vi "create_pb_arrayofarrays_synth_v2012.vi"(0 "PulseBlaster Array of Arrays":T12(array[cluster])=[{"Data Field"=0, "Delay"=0.005, "OP code"=8, "Output Bits"=[FALSE, TRUE, FALSE, FALSE, FALSE, FALSE, FALSE, FALSE, FALSE, FALSE, FALSE, FALSE, TRUE, FALSE, FALSE, FALSE, FALSE, FALSE, FALSE, FALSE, FALSE, FALSE, FALSE, FALSE], "String"="cool mot coils"}, {"Data Field"=300, "Delay"=0.000999, "OP code"=2, "Output Bits"=[TRUE, TRUE, TRUE, TRUE, FALSE, FALSE, TRUE, FALSE, FALSE, TRUE, FALSE, FALSE, TRUE, TRUE, FALSE, TRUE, TRUE, FALSE, FALSE, FALSE, FALSE, FALSE, FALSE, FALSE], "String"="mot load loop"}, {"Data Field"=1, "Delay"=1e-06, "OP code"=3, "Output Bits"=[TRUE, TRUE, TRUE, TRUE, FALSE, FALSE, TRUE, FALSE, FALSE, TRUE, FALSE, FALSE, TRUE, TRUE, FALSE, TRUE, TRUE, FALSE, FALSE, FALSE, FALSE, FALSE, FALSE, FALSE, FALSE], "String"=""}, {"Data Field"=0, "Delay"=0.001, "OP code"=0, "Output Bits"=[TRUE, TRUE, TRUE, TRUE, FALSE, FALSE, TRUE, FALSE, FALSE, TRUE, FALSE, FALSE, TRUE, TRUE, FALSE, TRUE, TRUE, FALSE, FALSE, FALSE, FALSE, FALSE, FALSE, FALSE], "String"=""}, {"Data Field"=2, "Delay"=0.000999, "OP code"=2, "Output Bits"=[TRUE, TRUE, TRUE, TRUE, FALSE, FALSE, TRUE, FALSE, FALSE, TRUE, FALSE, FALSE, TRUE, TRUE, FALSE, TRUE, TRUE, FALSE, FALSE, FALSE, FALSE, FALSE, FALSE, FALSE], "String"="mot decay loop"}, {"Data Field"=4, "Delay"=1e-06, "OP code"=3, "Output Bits"=[TRUE, TRUE, TRUE, TRUE, FALSE, FALSE, TRUE, FALSE, FALSE, TRUE, FALSE, FALSE, TRUE, TRUE, FALSE, TRUE, TRUE, FALSE, FALSE, FALSE, FALSE, FALSE, FALSE, FALSE], "String"=""}, {"Data Field"=0, "Delay"=0.000908, "OP code"=0, "Output Bits"=[TRUE, TRUE, TRUE, TRUE, FALSE, FALSE, TRUE, FALSE, FALSE, TRUE, FALSE, FALSE, TRUE, TRUE, FALSE, TRUE, TRUE, FALSE, FALSE, FALSE, FALSE, FALSE, FALSE, FALSE], "String"=""}, {"Data Field"=0, "Delay"=0.00865, "OP code"=0, "Output Bits"=[TRUE, TRUE, TRUE, TRUE, FALSE, FALSE, TRUE, FALSE, FALSE, TRUE, FALSE, FALSE, TRUE, TRUE, FALSE, TRUE, TRUE, FALSE, FALSE, FALSE, FALSE, FALSE, FALSE, FALSE], "String"=""}, {"Data Field"=0, "Delay"=0.004, "OP code"=0, "Output Bits"=[TRUE, TRUE, FALSE, TRUE, FALSE, FALSE, TRUE, FALSE, FALSE, TRUE, FALSE, FALSE, TRUE, TRUE, FALSE, TRUE, TRUE, FALSE, FALSE, FALSE, FALSE, FALSE, FALSE, FALSE], "String"=""}, {"Data Field"=0, "Delay"=0.0045, "OP code"=0, "Output Bits"=[TRUE, TRUE, FALSE, TRUE, FALSE, FALSE, TRUE, FALSE, FALSE, TRUE, FALSE, FALSE, TRUE, FALSE, FALSE, FALSE, TRUE, FALSE, FALSE, FALSE, FALSE, FALSE, FALSE, FALSE], "String"="Blue MOT Cooling Time"}, {"Data Field"=0, "Delay"=0.05, "OP code"=0, "Output Bits"=[FALSE, TRUE, FALSE, FALSE, FALSE, FALSE, FALSE, FALSE, FALSE, TRUE, TRUE, FALSE, TRUE, FALSE, FALSE, FALSE, FALSE, FALSE, FALSE, FALSE, FALSE, FALSE, FALSE, FALSE], "String"="Red MOT Cooling Time =="}, {"Data Field"=0, "Delay"=0.01, "OP code"=0, "Output Bits"=[FALSE, TRUE, FALSE, FALSE, FALSE, FALSE, FALSE, FALSE, FALSE, FALSE, FALSE, FALSE, FALSE, FALSE, FALSE, FALSE, FALSE, FALSE, FALSE, FALSE, FALSE, FALSE, FALSE, FALSE], "String"="PAS Beam with RED MOT            DELAY TIME BEFORE INTERAC"}, {"Data Field"=0, "Delay"=0.005, "OP code"=0, "Output Bits"=[FALSE, TRUE, FALSE, FALSE, FALSE, FALSE, FALSE, FALSE, FALSE, FALSE, FALSE, FALSE, FALSE, FALSE, FALSE, FALSE, TRUE, FALSE, FALSE, FALSE, FALSE, FALSE, FALSE, FALSE], "String"="image 12 delay (150n=90ndelay) INTERAC TIME"}, {"Data Field"=0, "Delay"=5e-05, "OP code"=0, "Output Bits"=[FALSE, TRUE, FALSE, FALSE, FALSE, FALSE, FALSE, FALSE, FALSE, FALSE, FALSE, FALSE, FALSE, FALSE, FALSE, FALSE, TRUE, TRUE, FALSE, FALSE, FALSE, FALSE, FALSE, FALSE], "String"="image beam on"}, {"Data Field"=0, "Delay"=0.0002, "OP code"=0, "Output Bits"=[FALSE, FALSE, FALSE, FALSE, FALSE, TRUE, FALSE, FALSE, FALSE, FALSE, FALSE, FALSE, FALSE, FALSE, FALSE, FALSE, TRUE, TRUE, FALSE, FALSE, FALSE, FALSE, FALSE, FALSE], "String"="camera minimum exposure time"}, {"Data Field"=0, "Delay"=0.07, "OP code"=0, "Output Bits"=[FALSE, FALSE, FALSE, FALSE, FALSE, FALSE, FALSE, FALSE, FALSE, FALSE, FALSE, FALSE, FALSE, FALSE, FALSE, FALSE, FALSE, TRUE, FALSE, FALSE, FALSE, FALSE, FALSE, FALSE], "String"="PixelFly Readout 1"}, {"Data Field"=0, "Delay"=0.005, "OP code"=0, "Output Bits"=[FALSE, FALSE, FALSE, FALSE, FALSE, FALSE, FALSE, FALSE, FALSE, FALSE, FALSE, FALSE, FALSE, FALSE, FALSE, FALSE, TRUE, TRUE, FALSE, FALSE, FALSE, FALSE, FALSE, FALSE], "String"="shutter opening time"}, {"Data Field"=0, "Delay"=0.0002, "OP code"=0, "Output Bits"=[FALSE, FALSE, FALSE, FALSE, FALSE, TRUE, FALSE, FALSE, FALSE, FALSE, FALSE, FALSE, FALSE, FALSE, FALSE, FALSE, TRUE, TRUE, FALSE, FALSE, FALSE, FALSE, FALSE, FALSE], "String"="Pixelfly exposure 2"}, {"Data Field"=0, "Delay"=0.07, "OP code"=0, "Output Bits"=[FALSE, FALSE, FALSE, FALSE, FALSE, FALSE, FALSE, FALSE, FALSE, FALSE, FALSE, FALSE, FALSE, FALSE, FALSE, FALSE, FALSE, FALSE, FALSE, FALSE, FALSE, FALSE, FALSE, FALSE], "String"="PixelFly readout 2"}, {"Data Field"=0, "Delay"=0.001, "OP code"=6, "Output Bits"=[FALSE, TRUE, TRUE, TRUE, FALSE, FALSE, FALSE, FALSE, FALSE, FALSE, FALSE, FALSE, TRUE, TRUE, FALSE, TRUE, FALSE, FALSE, FALSE, FALSE, FALSE, FALSE, FALSE, FALSE], "String"=""}] {"OP code" items=["Continue", "Stop", "Loop", "End Loop", "Jump", "Return", "Go To", "Long Delay", "Wait"]; "Delay" format="%.3p"}, 1 "6713 Write":dbl[](array[numeric])=[1.0, 4.0, 0.5, 6.5, 0.0, 9.58, 3.5, 0.5] format="%.3f", 2 "Arbitrary Waveform Array of Channels":T7(array[cluster])=[[{"AC Frequency (kHz)"=40.0, " Initial AC Ampl. (p-p/2)"=0.0, "Final AC Ampl."=0.0, "Initial DC Value"=-0.25, "Final DC Value"=0.05, "Constant"=165.3, "Gamma AC"=1.0, "String"="Channel 0 A", "Gamma DC"=1.0}, {"AC Frequency (kHz)"=40.0, " Initial AC Ampl. (p-p/2)"=0.0, "Final AC Ampl."=0.0, "Initial DC Value"=0.0, "Final DC Value"=0.0, "Constant"=165.2, "Gamma AC"=1.0, "String"="Channel 0 B", "Gamma DC"=1.0}, {"AC Frequency (kHz)"=40.0, " Initial AC Ampl. (p-p/2)"=0.0, "Final AC Ampl."=0.0, "Initial DC Value"=0.0, "Final DC Value"=0.0, "Constant"=163.20000000000002, "Gamma AC"=1.0, "String"="Channel 0 C", "Gamma DC"=1.0}], [{"AC Frequency (kHz)"=10.0, " Initial AC Ampl. (p-p/2)"=5.0, "Final AC Ampl."=0.0, "Initial DC Value"=0.2, "Final DC Value"=0.14, "Constant"=0.25, "Gamma AC"=1.0, "String"="Channel 1 A", "Gamma DC"=1.0}, {"AC Frequency (kHz)"=10.0, " Initial AC Ampl. (p-p/2)"=5.0, "Final AC Ampl."=0.0, "Initial DC Value"=0.1, "Final DC Value"=0.1, "Constant"=0.25, "Gamma AC"=1.0, "String"="Channel 1 B", "Gamma DC"=1.0}, {"AC Frequency (kHz)"=10.0, " Initial AC Ampl. (p-p/2)"=0.0, "Final AC Ampl."=0.0, "Initial DC Value"=0.0, "Final DC Value"=0.0, "Constant"=0.25, "Gamma AC"=1.0, "String"="Channel 1 C", "Gamma DC"=1.0}], [{"AC Frequency (kHz)"=10.0, " Initial AC Ampl. (p-p/2)"=0.0, "Final AC Ampl."=0.0, "Initial DC Value"=0.007, "Final DC Value"=0.04, "Constant"=0.0, "Gamma AC"=1.0, "String"="Channel 2 A", "Gamma DC"=1.0}, {"AC Frequency (kHz)"=10.0, " Initial AC Ampl. (p-p/2)"=0.0, "Final AC Ampl."=0.0, "Initial DC Value"=0.5, "Final DC Value"=0.5, "Constant"=0.0, "Gamma AC"=1.0, "String"="Channel 2 B", "Gamma DC"=1.0}, {"AC Frequency (kHz)"=10.0, " Initial AC Ampl. (p-p/2)"=0.0, "Final AC Ampl."=0.0, "Initial DC Value"=0.0, "Final DC Value"=0.0, "Constant"=0.0, "Gamma AC"=1.0, "String"="Channel 2 C", "Gamma DC"=1.0}], [{"AC Frequency (kHz)"=10.0, " Initial AC Ampl. (p-p/2)"=0.0, "Final AC Ampl."=0.0, "Initial DC Value"=1.0, "Final DC Value"=1.0, "Constant"=199.2, "Gamma AC"=1.0, "String"="Channel 3 A", "Gamma DC"=1.0}, {"AC Frequency (kHz)"=10.0, " Initial AC Ampl. (p-p/2)"=0.0, "Final AC Ampl."=0.0, "Initial DC Value"=1.0, "Final DC Value"=1.0, "Constant"=199.2, "Gamma AC"=1.0, "String"="Channel 3 B", "Gamma DC"=1.0}, {"AC Frequency (kHz)"=10.0, " Initial AC Ampl. (p-p/2)"=0.0, "Final AC Ampl."=0.0, "Initial DC Value"=1.0, "Final DC Value"=1.0, "Constant"=199.2, "Gamma AC"=1.0, "String"="Channel 3 C", "Gamma DC"=1.0}], [{"AC Frequency (kHz)"=10.0, " Initial AC Ampl. (p-p/2)"=0.0, "Final AC Ampl."=0.0, "Initial DC Value"=-0.1, "Final DC Value"=-0.04, "Constant"=199.2, "Gamma AC"=1.0, "String"="Channel 4 A", "Gamma DC"=1.0}, {"AC Frequency (kHz)"=10.0, " Initial AC Ampl. (p-p/2)"=0.0, "Final AC Ampl."=0.0, "Initial DC Value"=-0.1, "Final DC Value"=-0.04, "Constant"=199.2, "Gamma AC"=1.0, "String"="Channel 4 B", "Gamma DC"=1.0}, {"AC Frequency (kHz)"=10.0, " Initial AC Ampl. (p-p/2)"=0.0, "Final AC Ampl."=0.0, "Initial DC Value"=-0.1, "Final DC Value"=-0.04, "Constant"=199.2, "Gamma AC"=1.0, "String"="Channel 4 C", "Gamma DC"=1.0}], [{"AC Frequency (kHz)"=10.0, " Initial AC Ampl. (p-p/2)"=0.0, "Final AC Ampl."=0.0, "Initial DC Value"=-0.1, "Final DC Value"=-0.04, "Constant"=199.2, "Gamma AC"=1.0, "String"="Channel 5 A", "Gamma DC"=1.0}, {"AC Frequency (kHz)"=10.0, " Initial AC Ampl. (p-p/2)"=0.0, "Final AC Ampl."=0.0, "Initial DC Value"=-0.1, "Final DC Value"=-0.04, "Constant"=199.2, "Gamma AC"=1.0, "String"="Channel 5 B", "Gamma DC"=1.0}, {"AC Frequency (kHz)"=10.0, " Initial AC Ampl. (p-p/2)"=0.0, "Final AC Ampl."=0.0, "Initial DC Value"=-0.1, "Final DC Value"=-0.04, "Constant"=199.2, "Gamma AC"=1.0, "String"="Channel 5 C", "Gamma DC"=1.0}], [{"AC Frequency (kHz)"=10.0, " Initial AC Ampl. (p-p/2)"=0.0, "Final AC Ampl."=0.0, "Initial DC Value"=-0.1, "Final DC Value"=-0.04, "Constant"=199.2, "Gamma AC"=1.0, "String"="Channel 6 A", "Gamma DC"=1.0}, {"AC Frequency (kHz)"=10.0, " Initial AC Ampl. (p-p/2)"=0.0, "Final AC Ampl."=0.0, "Initial DC Value"=-0.1, "Final DC Value"=-0.04, "Constant"=199.2, "Gamma AC"=1.0, "String"="Channel 6 B", "Gamma DC"=1.0}, {"AC Frequency (kHz)"=10.0, " Initial AC Ampl. (p-p/2)"=0.0, "Final AC Ampl."=0.0, "Initial DC Value"=-0.1, "Final DC Value"=-0.04, "Constant"=199.2, "Gamma AC"=1.0, "String"="Channel 6 C", "Gamma DC"=1.0}], [{"AC Frequency (kHz)"=10.0, " Initial AC Ampl. (p-p/2)"=0.0, "Final AC Ampl."=0.0, "Initial DC Value"=-0.1, "Final DC Value"=-0.04, "Constant"=199.2, "Gamma AC"=1.0, "String"="Channel 7 A", "Gamma DC"=1.0}, {"AC Frequency (kHz)"=10.0, " Initial AC Ampl. (p-p/2)"=0.0, "Final AC Ampl."=0.0, "Initial DC Value"=-0.1, "Final DC Value"=-0.04, "Constant"=199.2, "Gamma AC"=1.0, "String"="Channel 7 B", "Gamma DC"=1.0}, {"AC Frequency (kHz)"=10.0, " Initial AC Ampl. (p-p/2)"=0.0, "Final AC Ampl."=0.0, "Initial DC Value"=-0.1, "Final DC Value"=-0.04, "Constant"=199.2, "Gamma AC"=1.0, "String"="Channel 7 C", "Gamma DC"=1.0}]] {"Gamma DC" format="%.2f"; "Gamma AC" format="%.2f"; "Constant" min=0.0 max=240.0 format="%.3f"; "Final DC Value" format="%.3f"; "Initial DC Value" format="%.3f"; "Final AC Ampl." format="%.3f"; "Initial AC Ampl. (p-p/2)" format="%.3f"; "AC Frequency (kHz)" format="%.2f"}, 3 "Interval Lengths (ms)":dbl[](array[numeric])=[55.0, 45.0, 1.0] format="%.3f", 4 "Intervals: ON or OFF?":bool[](array[boolean])=[TRUE, FALSE, FALSE], 5 "Waveform Change Parameters":T8={"Channel to Change"=0, "Interval to Change"=1, "Waveform Parameter\nto Change"=8} {"Waveform Parameter\nto Change" items=["Constant", "Initial DC", "Final DC", "Gamma DC", "AC Frequency", "Initial AC", "Gamma AC", "Final AC", "Interval Length"]; "Interval to Change" items=["A", "B", "C", "D", "E"]}, 6 "Arrays":T2={"Logarithmic Array"={"Initial Value"=1, "Fineness Factor"=1, "Number of Values"=10, "Generate Logarithmic\nArray?"=FALSE}, "Generated Array"={"Step Size"=-0.03, "Use generated\nDAC array values?"=FALSE, "Number of DAC Array\nValues to Generate"=67, "Initial Value for DAC"=[1.0]}} {"Generated Array"."Initial Value for DAC" format="%.2f"; "Generated Array"."Step Size" format="%.4f"}, 7 "Parameters to Change":T10={"PB parameter to change"=0, "Column of\nData to Change\n(0, 1, 2, ....)"=0, "Column of\nDelay to Change\n(0, 1, 2, ....)"=11, "6713 DAC Ch\nto Change"=7, "column for waveform\n(red mot cooling)"=10, "# of PB arrays"=1, "column for waveform\n(dipole trap loading)"=10, "Power\nSupply\nChannel"=1} {"Power\nSupply\nChannel" min=1 max=2; "PB parameter to change" min=0 max=8}, 8 "Synth":T3={"Table Mode On?"=FALSE, "Synth"=[{"AC Frequency (kHz)"=0.0, " Initial AC Ampl. (p-p/2)"=0.4, "Final AC Ampl."=0.4, "Frequency"=4.0, "Phase (rad)"=0.0, "Voltage (%)"=0.0, "Gamma AC"=1.0, "String"="Channel 0 A", "Blanck"=0.0}, {"AC Frequency (kHz)"=0.0, " Initial AC Ampl. (p-p/2)"=0.4, "Final AC Ampl."=0.4, "Frequency"=4.0, "Phase (rad)"=0.0, "Voltage (%)"=0.0, "Gamma AC"=1.0, "String"="Channel 0 B", "Blanck"=-0.3}, {"AC Frequency (kHz)"=0.0, " Initial AC Ampl. (p-p/2)"=0.4, "Final AC Ampl."=0.4, "Frequency"=1.0, "Phase (rad)"=0.0, "Voltage (%)"=2.0, "Gamma AC"=1.0, "String"="Channel 0 C", "Blanck"=0.0}, {"AC Frequency (kHz)"=0.0, " Initial AC Ampl. (p-p/2)"=0.4, "Final AC Ampl."=0.4, "Frequency"=7.0, "Phase (rad)"=1.0, "Voltage (%)"=2.0, "Gamma AC"=1.0, "String"="Channel 0 D", "Blanck"=1.4}, {"AC Frequency (kHz)"=0.0, " Initial AC Ampl. (p-p/2)"=0.0, "Final AC Ampl."=0.0, "Frequency"=0.6, "Phase (rad)"=1.0, "Voltage (%)"=1.0, "Gamma AC"=0.0, "String"="Channel 0 E", "Blanck"=0.2}]} {"Synth"."Blanck" format="%.2f"; "Synth"."Gamma AC" format="%.2f"; "Synth"."Voltage (%)" min=0.0 max=100.0 step=1.0; "Synth"."Phase (rad)" min=0.0 max=6.383118 format="%#_4f"; "Synth"."Frequency" min=0.0 max=10.0 format="%.7f"; "Synth"."Final AC Ampl." format="%.3f"; "Synth"."Initial AC Ampl. (p-p/2)" format="%.3f"; "Synth"."AC Frequency (kHz)" format="%.2f"}, 9 "dac offset":dbl format="%.2f", 11 "DAC Array":dbl[](array[numeric])=[0.05, 0.1, 0.15, 0.2, 0.25, 0.3, 0.35, 0.4, 0.45, 0.5, 9.6, 0.24, 0.26, 5.28, 0.3, 0.32, 0.34, 0.36, 0.38, 0.4, 5.0, 5.2, 5.4, 5.6, 5.8, 6.0, 6.2, 6.4, 6.6, 6.8, 7.0, 7.199999999999999, 7.4, 7.6, 7.800000000000001, 9.0, 6.8, 7.2, 7.6, 8.0, 8.4, 8.8, 9.0, 9.2, 9.4, 9.6, 9.8, 10.0, 0.4, 0.2, 0.0001, 0.0001, 0.0001, 0.0001, 0.0001, 0.0001, 0.0001, 0.0001, 0.0001, 0.0001, 0.0001, 0.0001, 0.0001, 0.0001, 0.0001, 0.0001, 0.0001, 0.0001, 0.0001, 0.0001, 0.0001, 0.0001, 0.0001, 0.0001, 0.0001, 0.0001, 0.0001, 0.0001, 0.0001, 0.0001, 0.0001, 0.0001, 0.0001, 0.0001, 0.0001, 0.0001, 0.0001, 0.0001, 0.0001, 0.0001, 0.0001, 0.0001, 0.0001, 0.0001, 0.0001, 0.0001, 0.0001, 0.0001, 0.0001, 0.0001, 0.0001, 0.0001, 0.0001, 0.0001, 0.0001, 0.0001, 0.0001, 0.0001, 0.0001, 0.0001, 0.0001, 0.0001, 0.0001, 0.0001, 0.0001, 0.0001, 0.0001, 0.0001, 0.0001, 0.0001, 0.0001, 0.0001, 0.0001, 0.0001, 0.0001, 0.0001, 0.0001, 0.0001, 0.0001, 0.0001, 0.0001, 0.0001, 0.0001, 0.0001, 0.0001, 0.0001, 0.0001, 0.0001, 0.0001, 0.0001, 0.0001, 0.0001, 0.0001, 0.0001, 0.0001, 0.0001, 0.0, 0.0, 0.0, 0.0, 0.0, 0.0, 0.0, 0.0, 0.0, 0.0, 0.0, 0.0, 0.0, 0.0, 0.0, 0.0, 0.0, 0.0, 0.0, 0.0, 0.0, 0.0, 0.0, 0.0, 0.0, 0.0, 0.0, 0.0, 0.0, 0.0, 0.0, 0.0, 0.0, 0.0, 0.0, 0.0, 0.0, 0.0, 0.0, 0.0, 0.0, 0.0, 0.0, 0.0, 0.0, 0.0, 0.0, 0.0, 0.0, 0.0, 0.0, 0.0, 0.0, 0.0, 0.0, 0.0, 0.0, 0.0, 0.0, 0.0, 0.0, 0.0, 0.0, 0.0, 0.0, 0.0, 0.0, 0.0, 0.0, 0.0, 0.0, 0.0, 0.0, 0.0, 0.0, 0.0, 0.0, 0.0, 0.0, 0.0, 0.0, 0.0, 0.0, 0.0, 0.0, 0.0, 0.0, 0.0, 0.0, 0.0, 0.0, 0.0, 0.0, 0.0, 0.0, 0.0, 0.0, 0.0, 0.0, 0.0, 0.0, 0.0, 0.0, 0.0, 0.0, 0.0, 0.0, 0.0, 0.0, 0.0, 0.0, 0.0, 0.0, 0.0, 0.0, 0.0, 0.0, 0.0, 0.0, 0.0, 0.0, 0.0, 0.0, 0.0, 0.0, 0.0, 0.0, 0.0, 0.0, 0.0, 0.0, 0.0, 0.0, 0.0, 0.0, 0.0, 0.0, 0.0, 0.0, 0.0, 0.0, 0.0, 0.0, 0.0, 0.0, 0.0, 0.0, 0.0, 0.0, 0.0, 0.0, 0.0, 0.0, 0.0, 0.0, 0.0, 0.0, 0.0, 0.0, 0.0, 0.0, 0.0, 0.0, 0.0, 0.0, 0.0, 0.0, 0.0, 0.0, 0.0, 0.0, 0.0, 0.0, 0.0, 0.0, 0.0, 0.0, 0.0, 0.0, 0.0, 0.0, 0.0, 0.0, 0.0, 0.0, 0.0, 0.0, 0.0, 0.0, 0.0, 0.0, 0.0, 0.0, 0.0, 0.0, 0.0, 0.0, 0.0, 0.0, 0.0, 0.0, 0.0, 0.0, 0.0, 0.0, 0.0, 0.0, 0.0, 0.0, 0.0, 0.0, 0.0, 0.0, 0.0, 0.0, 0.0, 0.0, 0.0, 0.0, 0.0, 0.0, 0.0, 0.0, 0.0, 0.0, 0.0, 0.0, 0.0, 0.0, 0.0, 0.0, 0.0, 0.0, 0.0, 0.0, 0.0, 0.0, 0.0, 0.0, 0.0, 0.0, 0.0, 0.0, 0.0, 0.0, 0.0, 0.0, 0.0, 0.0, 0.0, 0.0, 0.0, 0.0, 0.0, 0.0, 0.0, 0.0, 0.0, 0.0, 0.0, 0.0, 0.0, 0.0, 0.0, 0.0, 0.0, 0.0, 0.0, 0.0, 0.0, 0.0, 0.0, 0.0, 0.0, 0.0, 0.0, 0.0, 0.0, 0.0, 0.0, 0.0, 0.0, 0.0, 0.0, 0.0, 0.0, 0.0, 0.0, 0.0, 0.0, 0.0, 0.0, 0.0, 0.0, 0.0, 0.0, 0.0, 0.0, 0.0, 0.0, 0.0, 0.0, 0.0, 0.0, 0.0, 0.0, 0.0, 0.0, 0.0, 0.0, 0.0, 0.0, 0.0, 0.0, 0.0, 0.0, 0.0, 0.0, 0.0, 0.0, 0.0, 0.0, 0.0, 0.0, 0.0, 0.0, 0.0, 0.0, 0.0, 0.0, 0.0, 0.0, 0.0, 0.0, 0.0, 0.0, 0.0, 0.0, 0.0, 0.0, 0.0, 0.0, 0.0, 0.0, 0.0, 0.0, 0.0, 0.0, 0.0, 0.0, 0.0, 0.0, 0.0, 0.0, 0.0] caption="DAC array" format="%.3f", 13 "Delay Array":ext[](array[numeric])=[1.0, 5.0, 10.0, 15.0, 20.0, 17.0, 13.0, 8.0, 3.0, 25.0, 30.0, 40.0, 2.0, 10.0, 15.0, 20.0, 25.0, 30.0, 35.0, 50.0, 15.0, 14.0, 13.0, 12.0, 11.0, 10.0, 9.0, 8.0, 7.0, 6.0, 5.0, 4.0, 3.0, 2.0, 1.0, 2.0, 3.0, 4.0, 5.0, 6.0, 1.0, 4.0, 1.0, 8.0, 1.0, 12.0, 1.0, 16.0, 1.0, 4.0, 1.0, 8.0, 12.0, 1.0, 16.0, 1.0, 4.0, 1.0, 8.0, 1.0, 19.0, 1.0, 1.0, 1.0, 1.0, 1.0, 1.0, 1.0, 1.0, 1.0, 1.0, 1.0, 1.0, 1.0, 1.0, 1.0, 1.0, 1.0, 1.0, 1.0, 1.0, 1.0, 1.0, 1.0, 1.0, 1.0, 1.0, 1.0, 1.0, 1.0, 1.0, 1.0, 1.0, 1.0, 1.0, 1.0, 1.0, 1.0, 1.0, 1.0, 1.0, 1.0, 1.0, 1.0, 1.0, 1.0, 1.0, 1.0, 1.0, 1.0, 1.0, 1.0, 1.0, 1.0, 1.0, 1.0, 1.0, 1.0, 1.0, 1.0, 1.0, 1.0, 1.0, 1.0, 1.0, 1.0, 1.0, 1.0, 1.0, 1.0, 1.0, 1.0, 1.0, 1.0, 1.0, 1.0, 1.0, 1.0, 1.0, 0.00001, 0.00000100000000000000000004, 0.00000100000000000000000004, 0.00000100000000000000000004, 0.00000100000000000000000004, 0.00000100000000000000000004, 0.00000100000000000000000004, 0.0, 0.0, 0.0, 0.0, 0.0, 0.0, 0.0, 0.0, 0.0, 0.0, 0.0, 0.0, 0.0, 0.0, 0.0, 0.0, 0.0, 0.0, 0.0, 0.0, 0.0, 0.0, 0.0, 0.0, 0.0, 0.0, 0.0, 0.0, 0.0, 0.0, 0.0, 0.0, 0.0, 0.0, 0.0, 0.0, 0.0, 0.0, 0.0, 0.0, 0.0, 0.0, 0.0, 0.0, 0.0, 0.0, 0.0, 0.0, 0.0, 0.0, 0.0, 0.0, 0.0, 0.0, 0.0, 0.0, 0.0, 0.0, 0.0, 0.0, 0.0, 0.0, 0.0, 0.0, 0.0, 0.0, 0.0, 0.0, 0.0, 0.0, 0.0, 0.0, 0.0, 0.0, 0.0, 0.0, 0.0, 0.0, 0.0, 0.0, 0.0, 0.0, 0.0, 0.0, 0.0, 0.0, 0.0, 0.0, 0.0, 0.0, 0.0, 0.0, 0.0, 0.0, 0.0, 0.0, 0.0, 0.0, 0.0, 0.0, 0.0, 0.0, 0.0, 0.0, 0.0, 0.0, 0.0, 0.0, 0.0, 0.0, 0.0, 0.0, 0.0, 0.0, 0.0, 0.0, 0.0, 0.0, 0.0, 0.0, 0.0, 0.0, 0.0, 0.0, 0.0, 0.0, 0.0, 0.0, 0.0, 0.0, 0.0, 0.0, 0.0, 0.0, 0.0, 0.0, 0.0, 0.0, 0.0, 0.0, 0.0, 0.0, 0.0, 0.0, 0.0, 0.0, 0.0, 0.0, 0.0, 0.0, 0.0, 0.0, 0.0, 0.0, 0.0, 0.0, 0.0, 0.0, 0.0, 0.0, 0.0, 0.0, 0.0, 0.0, 0.0, 0.0, 0.0, 0.0, 0.0, 0.0, 0.0, 0.0, 0.0, 0.0, 0.0, 0.0, 0.0, 0.0, 0.0, 0.0, 0.0, 0.0, 0.0, 0.0, 0.0, 0.0, 0.0, 0.0, 0.0, 0.0, 0.0, 0.0, 0.0, 0.0, 0.0, 0.0, 0.0, 0.0, 0.0, 0.0, 0.0, 0.0, 0.0, 0.0, 0.0, 0.0, 0.0, 0.0, 0.0, 0.0, 0.0, 0.0, 0.0, 0.0, 0.0, 0.0, 0.0, 0.0, 0.0, 0.0, 0.0, 0.0, 0.0, 0.0, 0.0, 0.0, 0.0, 0.0, 0.0, 0.0, 0.0, 0.0, 0.0, 0.0, 0.0, 0.0, 0.0, 0.0, 0.0, 0.0, 0.0, 0.0, 0.0, 0.0, 0.0, 0.0, 0.0, 0.0, 0.0, 0.0, 0.0, 0.0, 0.0, 0.0, 0.0, 0.0, 0.0, 0.0, 0.0, 0.0, 0.0, 0.0, 0.0, 0.0, 0.0, 0.0, 0.0, 0.0, 0.0, 0.0, 0.0, 0.0, 0.0, 0.0, 0.0, 0.0, 0.0, 0.0, 0.0, 0.0, 0.0, 0.0, 0.0, 0.0, 0.0, 0.0, 0.0, 0.0, 0.0, 0.0, 0.0, 0.0, 0.0, 0.0, 0.0, 0.0, 0.0, 0.0, 0.0, 0.0, 0.0, 0.0, 0.0, 0.0, 0.0, 0.0, 0.0, 0.0, 0.0, 0.0, 0.0, 0.0, 0.0, 0.0, 0.0, 0.0, 0.0, 0.0, 0.0, 0.0, 0.0, 0.0, 0.0, 0.0, 0.0, 0.0, 0.0, 0.0, 0.0, 0.0, 0.0, 0.0, 0.0, 0.0, 0.0, 0.0, 0.0, 0.0, 0.0, 0.0, 0.0, 0.0, 0.0, 0.0, 0.0, 0.0, 0.0, 0.0, 0.0, 0.0, 0.0, 0.0, 0.0, 0.0, 0.0] caption="Array of \nimage delay \nfields(in ms)" format="%.5f", 14 "Power Supply Controls":T5={"+6V output Voltage"=6.0, "+6V output Current"=1.812, "+25V output Voltage"=25.0, "+25V output Current"=0.241} {"+25V output Current" format="%.3f"; "+25V output Voltage" format="%.3f"; "+6V output Current" format="%.3f"; "+6V output Voltage" format="%.3f"}, 15 "Data Array":i16[](array[numeric])=[2, 4, 6, 7, 10, 14, 20, 25, 38, 40, 50, 70, 87, 120, 140, 160, 180, 200, 250, 300, 10, 7, 8, 9, 15, 16, 36, 41, 80, 145, 205, 19, 58, 49, 29, 199, 160, 151, 148, 33, 34, 34, 36, 37, 38, 1, 1, 1, 1, 1, 1, 1, 1, 1, 1, 1, 1, 1, 1, 1, 1, 1, 1, 1, 1, 1, 1, 1, 1, 1, 1, 1, 1, 1, 1, 1, 1, 1, 1, 1, 1, 1, 1, 1, 1, 1, 1, 1, 1, 1, 1, 1, 1, 1, 1, 1, 1, 1, 1, 1, 1, 1, 1, 1, 1, 1, 1, 1, 1, 1, 1, 1, 1, 1, 1, 1, 1, 1, 1, 1, 1, 1, 1, 1, 1, 1, 1, 1, 1, 1, 1, 1, 1, 1, 1, 1, 1, 1, 1, 1, 1, 1, 1, 1, 1, 1, 1, 1, 1, 1, 1, 1, 1, 1, 1, 1, 1, 1, 1, 0, 0, 0, 0, 0, 0, 0, 0, 0, 0, 0, 0, 0, 0, 0, 0, 0, 0, 0, 0, 0, 0, 0, 0, 0, 0, 0, 0, 0, 0, 0, 0, 0, 0, 0, 0, 0, 0, 0, 0, 0, 0, 0, 0, 0, 0, 0, 0, 0, 0, 0, 0, 0, 0, 0, 0, 0, 0, 0, 0, 0, 0, 0, 0, 0, 0, 0, 0, 0, 0, 0, 0, 0, 0, 0, 0, 0, 0, 0, 0, 0, 0, 0, 0, 0, 0, 0, 0, 0, 0, 0, 0, 0, 0, 0, 0, 0, 0, 0, 0, 0, 0, 0, 0, 0, 0, 0, 0, 0, 0, 0, 0, 0, 0, 0, 0, 0, 0, 0, 0, 0, 0, 0, 0, 0, 0, 0, 0, 0, 0, 0, 0, 0, 0, 0, 0, 0, 0, 0, 0, 0, 0, 0, 0, 0, 0, 0, 0, 0, 0, 0, 0, 0, 0, 0, 0, 0, 0, 0, 0, 0, 0, 0, 0, 0, 0, 0, 0, 0, 0, 0, 0, 0, 0, 0, 0, 0, 0, 0, 0, 0, 0, 0, 0, 0, 0, 0, 0, 0, 0, 0, 0, 0, 0, 0, 0, 0, 0, 0, 0, 0, 0, 0, 0, 0, 0, 0, 0, 0, 0, 0, 0, 0, 0, 0, 0, 0, 0, 0, 0, 0, 0, 0, 0, 0, 0, 0, 0, 0, 0, 0, 0, 0, 0, 0, 0, 0, 0, 0, 0, 0, 0, 0, 0, 0, 0, 0, 0, 0, 0, 0, 0, 0, 0, 0, 0, 0, 0, 0, 0, 0, 0, 0, 0, 0, 0, 0, 0, 0, 0, 0, 0, 0, 0, 0, 0, 0, 0, 0, 0, 0, 0, 0, 0, 0, 0, 0, 0, 0, 0, 0, 0, 0, 0, 0, 0, 0, 0, 0, 0, 0, 0, 0, 0, 0, 0, 0, 0, 0, 0, 0, 0, 0, 0, 0, 0, 0, 0, 0, 0, 0, 0, 0, 0, 0, 0, 0, 0, 0, 0, 0, 0, 0, 0, 0, 0, 0, 0, 0, 0, 0, 0] caption="Array of hold \ndata fields\n(number of \ndelay loops)", 17 "Waveform array":dbl[](array[numeric])=[50.0, 100.0, 150.0, 200.0, 250.0, 300.0, 275.0, 225.0, 175.0, 125.0, 75.0, 325.0, 164.7, 165.9, 165.6, 165.3, 166.8, 166.5, 166.2, 167.1, 167.4, 167.7, 168.0, 168.3, 168.6, 168.9, 169.2, 169.5, 169.8, 170.1, 170.4, 170.7, 171.0, 160.0, 160.3, 160.6, 160.9, 151.0, 148.0, 33.0, 35.0, 38.0, 39.0, 0.0001, 0.0001, 0.0001, 0.0001, 0.0001, 0.0001, 0.0001, 0.0001, 0.0001, 0.0001, 0.0001, 0.0001, 0.0001, 0.0001, 0.0001, 0.0001, 0.0001, 0.0001, 0.0001, 0.0001, 0.0001, 0.0001, 0.0001, 0.0001, 0.0001, 0.0001, 0.0001, 0.0001, 0.0001, 0.0001, 0.0001, 0.0001, 0.0001, 0.0001, 0.0001, 0.0001, 0.0001, 0.0001, 0.0001, 0.0001, 0.0001, 0.0001, 0.0001, 0.0001, 0.0001, 0.0001, 0.0001, 0.0001, 0.0001, 0.0001, 0.0001, 0.0001, 0.0001, 0.0001, 0.0001, 0.0001, 0.0001, 0.0001, 0.0001, 0.0001, 0.0001, 0.0001, 0.0001, 0.0001, 0.0001, 0.0001, 0.0001, 0.0001, 0.0001, 0.0001, 0.0001, 0.0001, 0.0001, 0.0001, 0.0001, 0.0001, 0.0001, 0.0001, 0.0001, 0.0001, 0.0001, 0.0001, 0.0001, 0.0001, 0.0001, 0.0001, 0.0001, 0.0001, 0.0001, 0.0001, 0.0001, 0.0001, 0.0001, 0.0001, 0.0001, 0.0001, 0.0001, 0.0001, 0.0001, 0.0001, 0.0001, 0.0001, 0.0001, 0.0001, 0.0001, 0.0001, 0.0001, 0.0001, 0.0, 0.0, 0.0, 0.0, 0.0, 0.0, 0.0, 0.0, 0.0, 0.0, 0.0, 0.0, 0.0, 0.0, 0.0, 0.0, 0.0, 0.0, 0.0, 0.0, 0.0, 0.0, 0.0, 0.0, 0.0, 0.0, 0.0, 0.0, 0.0, 0.0, 0.0, 0.0, 0.0, 0.0, 0.0, 0.0, 0.0, 0.0, 0.0, 0.0, 0.0, 0.0, 0.0, 0.0, 0.0, 0.0, 0.0, 0.0, 0.0, 0.0, 0.0, 0.0, 0.0, 0.0, 0.0, 0.0, 0.0, 0.0, 0.0, 0.0, 0.0, 0.0, 0.0, 0.0, 0.0, 0.0, 0.0, 0.0, 0.0, 0.0, 0.0, 0.0, 0.0, 0.0, 0.0, 0.0, 0.0, 0.0, 0.0, 0.0, 0.0, 0.0, 0.0, 0.0, 0.0, 0.0, 0.0, 0.0, 0.0, 0.0, 0.0, 0.0, 0.0, 0.0, 0.0, 0.0, 0.0, 0.0, 0.0, 0.0, 0.0, 0.0, 0.0, 0.0, 0.0, 0.0, 0.0, 0.0, 0.0, 0.0, 0.0, 0.0, 0.0, 0.0, 0.0, 0.0, 0.0, 0.0, 0.0, 0.0, 0.0, 0.0, 0.0, 0.0, 0.0, 0.0, 0.0, 0.0, 0.0, 0.0, 0.0, 0.0, 0.0, 0.0, 0.0, 0.0, 0.0, 0.0, 0.0, 0.0, 0.0, 0.0, 0.0, 0.0, 0.0, 0.0, 0.0, 0.0, 0.0, 0.0, 0.0, 0.0, 0.0, 0.0, 0.0, 0.0, 0.0, 0.0, 0.0, 0.0, 0.0, 0.0, 0.0, 0.0, 0.0, 0.0, 0.0, 0.0, 0.0, 0.0, 0.0, 0.0, 0.0, 0.0, 0.0, 0.0, 0.0, 0.0, 0.0, 0.0, 0.0, 0.0, 0.0, 0.0, 0.0, 0.0, 0.0, 0.0, 0.0, 0.0, 0.0, 0.0, 0.0, 0.0, 0.0, 0.0, 0.0, 0.0, 0.0, 0.0, 0.0, 0.0, 0.0, 0.0, 0.0, 0.0, 0.0, 0.0, 0.0, 0.0, 0.0, 0.0, 0.0, 0.0, 0.0, 0.0, 0.0, 0.0, 0.0, 0.0, 0.0, 0.0, 0.0, 0.0, 0.0, 0.0, 0.0, 0.0, 0.0, 0.0, 0.0, 0.0, 0.0, 0.0, 0.0, 0.0, 0.0, 0.0, 0.0, 0.0, 0.0, 0.0, 0.0, 0.0, 0.0, 0.0, 0.0, 0.0, 0.0, 0.0, 0.0, 0.0, 0.0, 0.0, 0.0, 0.0, 0.0, 0.0, 0.0, 0.0, 0.0, 0.0, 0.0, 0.0, 0.0, 0.0, 0.0, 0.0, 0.0, 0.0, 0.0, 0.0, 0.0, 0.0, 0.0, 0.0, 0.0, 0.0, 0.0, 0.0, 0.0, 0.0, 0.0, 0.0, 0.0, 0.0, 0.0, 0.0, 0.0, 0.0, 0.0, 0.0, 0.0, 0.0, 0.0, 0.0, 0.0, 0.0, 0.0, 0.0, 0.0, 0.0, 0.0, 0.0, 0.0, 0.0, 0.0, 0.0, 0.0, 0.0, 0.0, 0.0, 0.0, 0.0, 0.0, 0.0, 0.0, 0.0, 0.0, 0.0, 0.0, 0.0, 0.0, 0.0, 0.0, 0.0, 0.0, 0.0, 0.0, 0.0, 0.0, 0.0, 0.0, 0.0, 0.0, 0.0, 0.0, 0.0, 0.0, 0.0, 0.0, 0.0, 0.0, 0.0, 0.0, 0.0, 0.0, 0.0, 0.0, 0.0] caption="waveform array\nparameter to change" format="%.3f", 19 "Adiabatic Loading Waveform":T7(array[cluster])=[[{"AC Frequency (kHz)"=0.0, " Initial AC Ampl. (p-p/2)"=0.0, "Final AC Ampl."=0.0, "Initial DC Value"=7.0, "Final DC Value"=1.0, "Constant"=2.0, "Gamma AC"=1.0, "String"="Channel 0 A", "Gamma DC"=1.0}, {"AC Frequency (kHz)"=40.0, " Initial AC Ampl. (p-p/2)"=0.0, "Final AC Ampl."=0.0, "Initial DC Value"=-0.6, "Final DC Value"=-0.6, "Constant"=165.8, "Gamma AC"=1.0, "String"="Channel 0 B", "Gamma DC"=1.0}, {"AC Frequency (kHz)"=40.0, " Initial AC Ampl. (p-p/2)"=0.0, "Final AC Ampl."=0.0, "Initial DC Value"=0.0, "Final DC Value"=0.0, "Constant"=162.7, "Gamma AC"=1.0, "String"="Channel 0 C", "Gamma DC"=1.0}], [{"AC Frequency (kHz)"=10.0, " Initial AC Ampl. (p-p/2)"=5.0, "Final AC Ampl."=0.0, "Initial DC Value"=0.2, "Final DC Value"=0.16, "Constant"=0.25, "Gamma AC"=1.0, "String"="Channel 1 A", "Gamma DC"=1.0}, {"AC Frequency (kHz)"=10.0, " Initial AC Ampl. (p-p/2)"=5.0, "Final AC Ampl."=0.0, "Initial DC Value"=0.16, "Final DC Value"=0.16, "Constant"=0.25, "Gamma AC"=1.0, "String"="Channel 1 B", "Gamma DC"=1.0}, {"AC Frequency (kHz)"=10.0, " Initial AC Ampl. (p-p/2)"=0.0, "Final AC Ampl."=0.0, "Initial DC Value"=0.0, "Final DC Value"=0.0, "Constant"=0.25, "Gamma AC"=1.0, "String"="Channel 1 C", "Gamma DC"=1.0}], [{"AC Frequency (kHz)"=10.0, " Initial AC Ampl. (p-p/2)"=0.0, "Final AC Ampl."=0.0, "Initial DC Value"=0.007, "Final DC Value"=0.06, "Constant"=0.0, "Gamma AC"=1.0, "String"="Channel 2 A", "Gamma DC"=1.0}, {"AC Frequency (kHz)"=10.0, " Initial AC Ampl. (p-p/2)"=0.0, "Final AC Ampl."=0.0, "Initial DC Value"=0.06, "Final DC Value"=0.06, "Constant"=0.0, "Gamma AC"=1.0, "String"="Channel 2 B", "Gamma DC"=1.0}, {"AC Frequency (kHz)"=10.0, " Initial AC Ampl. (p-p/2)"=0.0, "Final AC Ampl."=0.0, "Initial DC Value"=0.0, "Final DC Value"=0.0, "Constant"=0.0, "Gamma AC"=1.0, "String"="Channel 2 C", "Gamma DC"=1.0}], [{"AC Frequency (kHz)"=10.0, " Initial AC Ampl. (p-p/2)"=0.0, "Final AC Ampl."=0.0, "Initial DC Value"=1.0, "Final DC Value"=1.0, "Constant"=199.2, "Gamma AC"=1.0, "String"="Channel 3 A", "Gamma DC"=1.0}, {"AC Frequency (kHz)"=10.0, " Initial AC Ampl. (p-p/2)"=0.0, "Final AC Ampl."=0.0, "Initial DC Value"=1.0, "Final DC Value"=1.0, "Constant"=199.2, "Gamma AC"=1.0, "String"="Channel 3 B", "Gamma DC"=1.0}, {"AC Frequency (kHz)"=10.0, " Initial AC Ampl. (p-p/2)"=0.0, "Final AC Ampl."=0.0, "Initial DC Value"=1.0, "Final DC Value"=1.0, "Constant"=199.2, "Gamma AC"=1.0, "String"="Channel 3 C", "Gamma DC"=1.0}], [{"AC Frequency (kHz)"=10.0, " Initial AC Ampl. (p-p/2)"=0.0, "Final AC Ampl."=0.0, "Initial DC Value"=-0.1, "Final DC Value"=-0.04, "Constant"=199.2, "Gamma AC"=1.0, "String"="Channel 4 A", "Gamma DC"=1.0}, {"AC Frequency (kHz)"=10.0, " Initial AC Ampl. (p-p/2)"=0.0, "Final AC Ampl."=0.0, "Initial DC Value"=-0.1, "Final DC Value"=-0.04, "Constant"=199.2, "Gamma AC"=1.0, "String"="Channel 4 B", "Gamma DC"=1.0}, {"AC Frequency (kHz)"=10.0, " Initial AC Ampl. (p-p/2)"=0.0, "Final AC Ampl."=0.0, "Initial DC Value"=-0.1, "Final DC Value"=-0.04, "Constant"=199.2, "Gamma AC"=1.0, "String"="Channel 4 C", "Gamma DC"=1.0}], [{"AC Frequency (kHz)"=10.0, " Initial AC Ampl. (p-p/2)"=0.0, "Final AC Ampl."=0.0, "Initial DC Value"=-0.1, "Final DC Value"=-0.04, "Constant"=199.2, "Gamma AC"=1.0, "String"="Channel 5 A", "Gamma DC"=1.0}, {"AC Frequency (kHz)"=10.0, " Initial AC Ampl. (p-p/2)"=0.0, "Final AC Ampl."=0.0, "Initial DC Value"=-0.1, "Final DC Value"=-0.04, "Constant"=199.2, "Gamma AC"=1.0, "String"="Channel 5 B", "Gamma DC"=1.0}, {"AC Frequency (kHz)"=10.0, " Initial AC Ampl. (p-p/2)"=0.0, "Final AC Ampl."=0.0, "Initial DC Value"=-0.1, "Final DC Value"=-0.04, "Constant"=199.2, "Gamma AC"=1.0, "String"="Channel 5 C", "Gamma DC"=1.0}], [{"AC Frequency (kHz)"=10.0, " Initial AC Ampl. (p-p/2)"=0.0, "Final AC Ampl."=0.0, "Initial DC Value"=-0.1, "Final DC Value"=-0.04, "Constant"=199.2, "Gamma AC"=1.0, "String"="Channel 6 A", "Gamma DC"=1.0}, {"AC Frequency (kHz)"=10.0, " Initial AC Ampl. (p-p/2)"=0.0, "Final AC Ampl."=0.0, "Initial DC Value"=-0.1, "Final DC Value"=-0.04, "Constant"=199.2, "Gamma AC"=1.0, "String"="Channel 6 B", "Gamma DC"=1.0}, {"AC Frequency (kHz)"=10.0, " Initial AC Ampl. (p-p/2)"=0.0, "Final AC Ampl."=0.0, "Initial DC Value"=-0.1, "Final DC Value"=-0.04, "Constant"=199.2, "Gamma AC"=1.0, "String"="Channel 6 C", "Gamma DC"=1.0}], [{"AC Frequency (kHz)"=10.0, " Initial AC Ampl. (p-p/2)"=0.0, "Final AC Ampl."=0.0, "Initial DC Value"=-0.1, "Final DC Value"=-0.04, "Constant"=199.2, "Gamma AC"=1.0, "String"="Channel 7 A", "Gamma DC"=1.0}, {"AC Frequency (kHz)"=10.0, " Initial AC Ampl. (p-p/2)"=0.0, "Final AC Ampl."=0.0, "Initial DC Value"=-0.1, "Final DC Value"=-0.04, "Constant"=199.2, "Gamma AC"=1.0, "String"="Channel 7 B", "Gamma DC"=1.0}, {"AC Frequency (kHz)"=10.0, " Initial AC Ampl. (p-p/2)"=0.0, "Final AC Ampl."=0.0, "Initial DC Value"=-0.1, "Final DC Value"=-0.04, "Constant"=199.2, "Gamma AC"=1.0, "String"="Channel 7 C", "Gamma DC"=1.0}]] {"Gamma DC" format="%.2f"; "Gamma AC" format="%.2f"; "Constant" min=0.0 max=240.0 format="%.2f"; "Final DC Value" format="%.3f"; "Initial DC Value" format="%.3f"; "Final AC Ampl." format="%.3f"; "Initial AC Ampl. (p-p/2)" format="%.3f"; "AC Frequency (kHz)" format="%.2f"}, 25 "ODT Interval Lengths (ms)":dbl[](array[numeric])=[50.0, 255.0, 50.0] format="%.3f", 26 "ODT Intervals: ON or OFF?":bool[](array[boolean])=[TRUE, TRUE, FALSE]) -> (10 "changed\nquantity":dbl[](array[numeric]), 12 "SynthOut":T1={"Table Mode On"=FALSE, "SynthesizerArrayofArrays"=[[{"AC Frequency (kHz)"=0.0, " Initial AC Ampl. (p-p/2)"=0.4, "Final AC Ampl."=0.4, "Frequency"=4.0, "Phase"=0.0, "Voltage"=0.0, "Gamma AC"=1.0, "String"="Channel 0 A", "Blanck"=0.0}, {"AC Frequency (kHz)"=0.0, " Initial AC Ampl. (p-p/2)"=0.4, "Final AC Ampl."=0.4, "Frequency"=4.0, "Phase"=0.0, "Voltage"=0.0, "Gamma AC"=1.0, "String"="Channel 0 B", "Blanck"=-0.3}, {"AC Frequency (kHz)"=0.0, " Initial AC Ampl. (p-p/2)"=0.4, "Final AC Ampl."=0.4, "Frequency"=1.0, "Phase"=0.0, "Voltage"=2.0, "Gamma AC"=1.0, "String"="Channel 0 C", "Blanck"=0.0}, {"AC Frequency (kHz)"=0.0, " Initial AC Ampl. (p-p/2)"=0.4, "Final AC Ampl."=0.4, "Frequency"=7.0, "Phase"=1.0, "Voltage"=2.0, "Gamma AC"=1.0, "String"="Channel 0 D", "Blanck"=1.4}, {"AC Frequency (kHz)"=0.0, " Initial AC Ampl. (p-p/2)"=0.0, "Final AC Ampl."=0.0, "Frequency"=0.6, "Phase"=1.0, "Voltage"=1.0, "Gamma AC"=0.0, "String"="Channel 0 E", "Blanck"=0.2}]]} {"SynthesizerArrayofArrays"."Blanck" format="%.2f"; "SynthesizerArrayofArrays"."Gamma AC" format="%.2f"; "SynthesizerArrayofArrays"."Voltage" min=0.0 max=100.0 step=1.0; "SynthesizerArrayofArrays"."Phase" min=0.0 max=6.383118 format="%#_4f"; "SynthesizerArrayofArrays"."Frequency" min=0.0 max=10.0 format="%.7f"; "SynthesizerArrayofArrays"."Final AC Ampl." format="%.3f"; "SynthesizerArrayofArrays"."Initial AC Ampl. (p-p/2)" format="%.3f"; "SynthesizerArrayofArrays"."AC Frequency (kHz)" format="%.2f"}, 16 "Power Supply Array":T4(array[cluster]), 18 "Adiabatic Loading Waveform\nArray of Channels":T6(array[cluster]), 20 "PB Array of Arrays":T11(array[cluster]), 21 "Array of 6713\nValues":dbl[][](array[numeric]), 22 "ArbWaveform Array\nof Channels":T6(array[cluster]), 23 "ArbWaveform Interval Lengths":dbl[][](array[numeric]), 24 "Generated\nDAC Array":dbl[](array[numeric])=[1.0, 0.97, 0.94, 0.9099999999999999, 0.8799999999999999, 0.8499999999999999, 0.8199999999999998, 0.7899999999999998, 0.7599999999999998, 0.7299999999999998, 0.6999999999999997, 0.6699999999999997, 0.6399999999999997, 0.6099999999999997, 0.5799999999999996, 0.5499999999999996, 0.5199999999999996, 0.48999999999999955, 0.4599999999999995, 0.4299999999999995, 0.39999999999999947, 0.36999999999999944, 0.3399999999999994, 0.3099999999999994, 0.27999999999999936, 0.24999999999999936, 0.21999999999999936, 0.18999999999999936, 0.15999999999999936, 0.12999999999999937, 0.09999999999999937, 0.06999999999999937, 0.03999999999999937, 0.00999999999999937, -0.02000000000000063, -0.05000000000000063, -0.08000000000000063, -0.11000000000000063, -0.14000000000000062, -0.17000000000000062, -0.20000000000000062, -0.23000000000000062, -0.2600000000000006, -0.2900000000000006, -0.3200000000000006, -0.35000000000000064, -0.38000000000000067, -0.4100000000000007, -0.4400000000000007, -0.47000000000000075, -0.5000000000000008, -0.5300000000000008, -0.5600000000000008, -0.5900000000000009, -0.6200000000000009, -0.6500000000000009, -0.6800000000000009, -0.710000000000001, -0.740000000000001, -0.770000000000001, -0.800000000000001, -0.8300000000000011, -0.8600000000000011, -0.8900000000000011, -0.9200000000000012, -0.9500000000000012, -0.9800000000000012, -1.0100000000000011] format="%.4f", 27 "output params to change":T9)   [LabVIEW 2013]
uses:
  Instance           2 43Saved   create_pb_arrayofarrays_synth_v2012 .vi
panel:
  in  "Case Constant\n(See Context Help)":bool=TRUE
  in  "SynthOutTemplate":T1={"Table Mode On"=FALSE, "SynthesizerArrayofArrays"=[[{"AC Frequency (kHz)"=0.0, " Initial AC Ampl. (p-p/2)"=0.4, "Final AC Ampl."=0.4, "Frequency"=4.0, "Phase"=0.0, "Voltage"=0.0, "Gamma AC"=1.0, "String"="Channel 0 A", "Blanck"=0.0}, {"AC Frequency (kHz)"=0.0, " Initial AC Ampl. (p-p/2)"=0.4, "Final AC Ampl."=0.4, "Frequency"=4.0, "Phase"=0.0, "Voltage"=0.0, "Gamma AC"=1.0, "String"="Channel 0 B", "Blanck"=-0.3}, {"AC Frequency (kHz)"=0.0, " Initial AC Ampl. (p-p/2)"=0.4, "Final AC Ampl."=0.4, "Frequency"=1.0, "Phase"=0.0, "Voltage"=2.0, "Gamma AC"=1.0, "String"="Channel 0 C", "Blanck"=0.0}, {"AC Frequency (kHz)"=0.0, " Initial AC Ampl. (p-p/2)"=0.4, "Final AC Ampl."=0.4, "Frequency"=7.0, "Phase"=1.0, "Voltage"=2.0, "Gamma AC"=1.0, "String"="Channel 0 D", "Blanck"=1.4}, {"AC Frequency (kHz)"=0.0, " Initial AC Ampl. (p-p/2)"=0.0, "Final AC Ampl."=0.0, "Frequency"=0.6, "Phase"=1.0, "Voltage"=1.0, "Gamma AC"=0.0, "String"="Channel 0 E", "Blanck"=0.2}]]} {"SynthesizerArrayofArrays"."Blanck" format="%.2f"; "SynthesizerArrayofArrays"."Gamma AC" format="%.2f"; "SynthesizerArrayofArrays"."Voltage" min=0.0 max=100.0 step=1.0; "SynthesizerArrayofArrays"."Phase" min=0.0 max=6.383118 format="%#_4f"; "SynthesizerArrayofArrays"."Frequency" min=0.0 max=10.0 format="%.7f"; "SynthesizerArrayofArrays"."Final AC Ampl." format="%.3f"; "SynthesizerArrayofArrays"."Initial AC Ampl. (p-p/2)" format="%.3f"; "SynthesizerArrayofArrays"."AC Frequency (kHz)" format="%.2f"}
  out "red mot cooling time":dbl[](array[numeric])
  in  "Front Panel Item\n(Box of Labels)":i32(listbox)=12
  # "(smaller makes\nblue)"
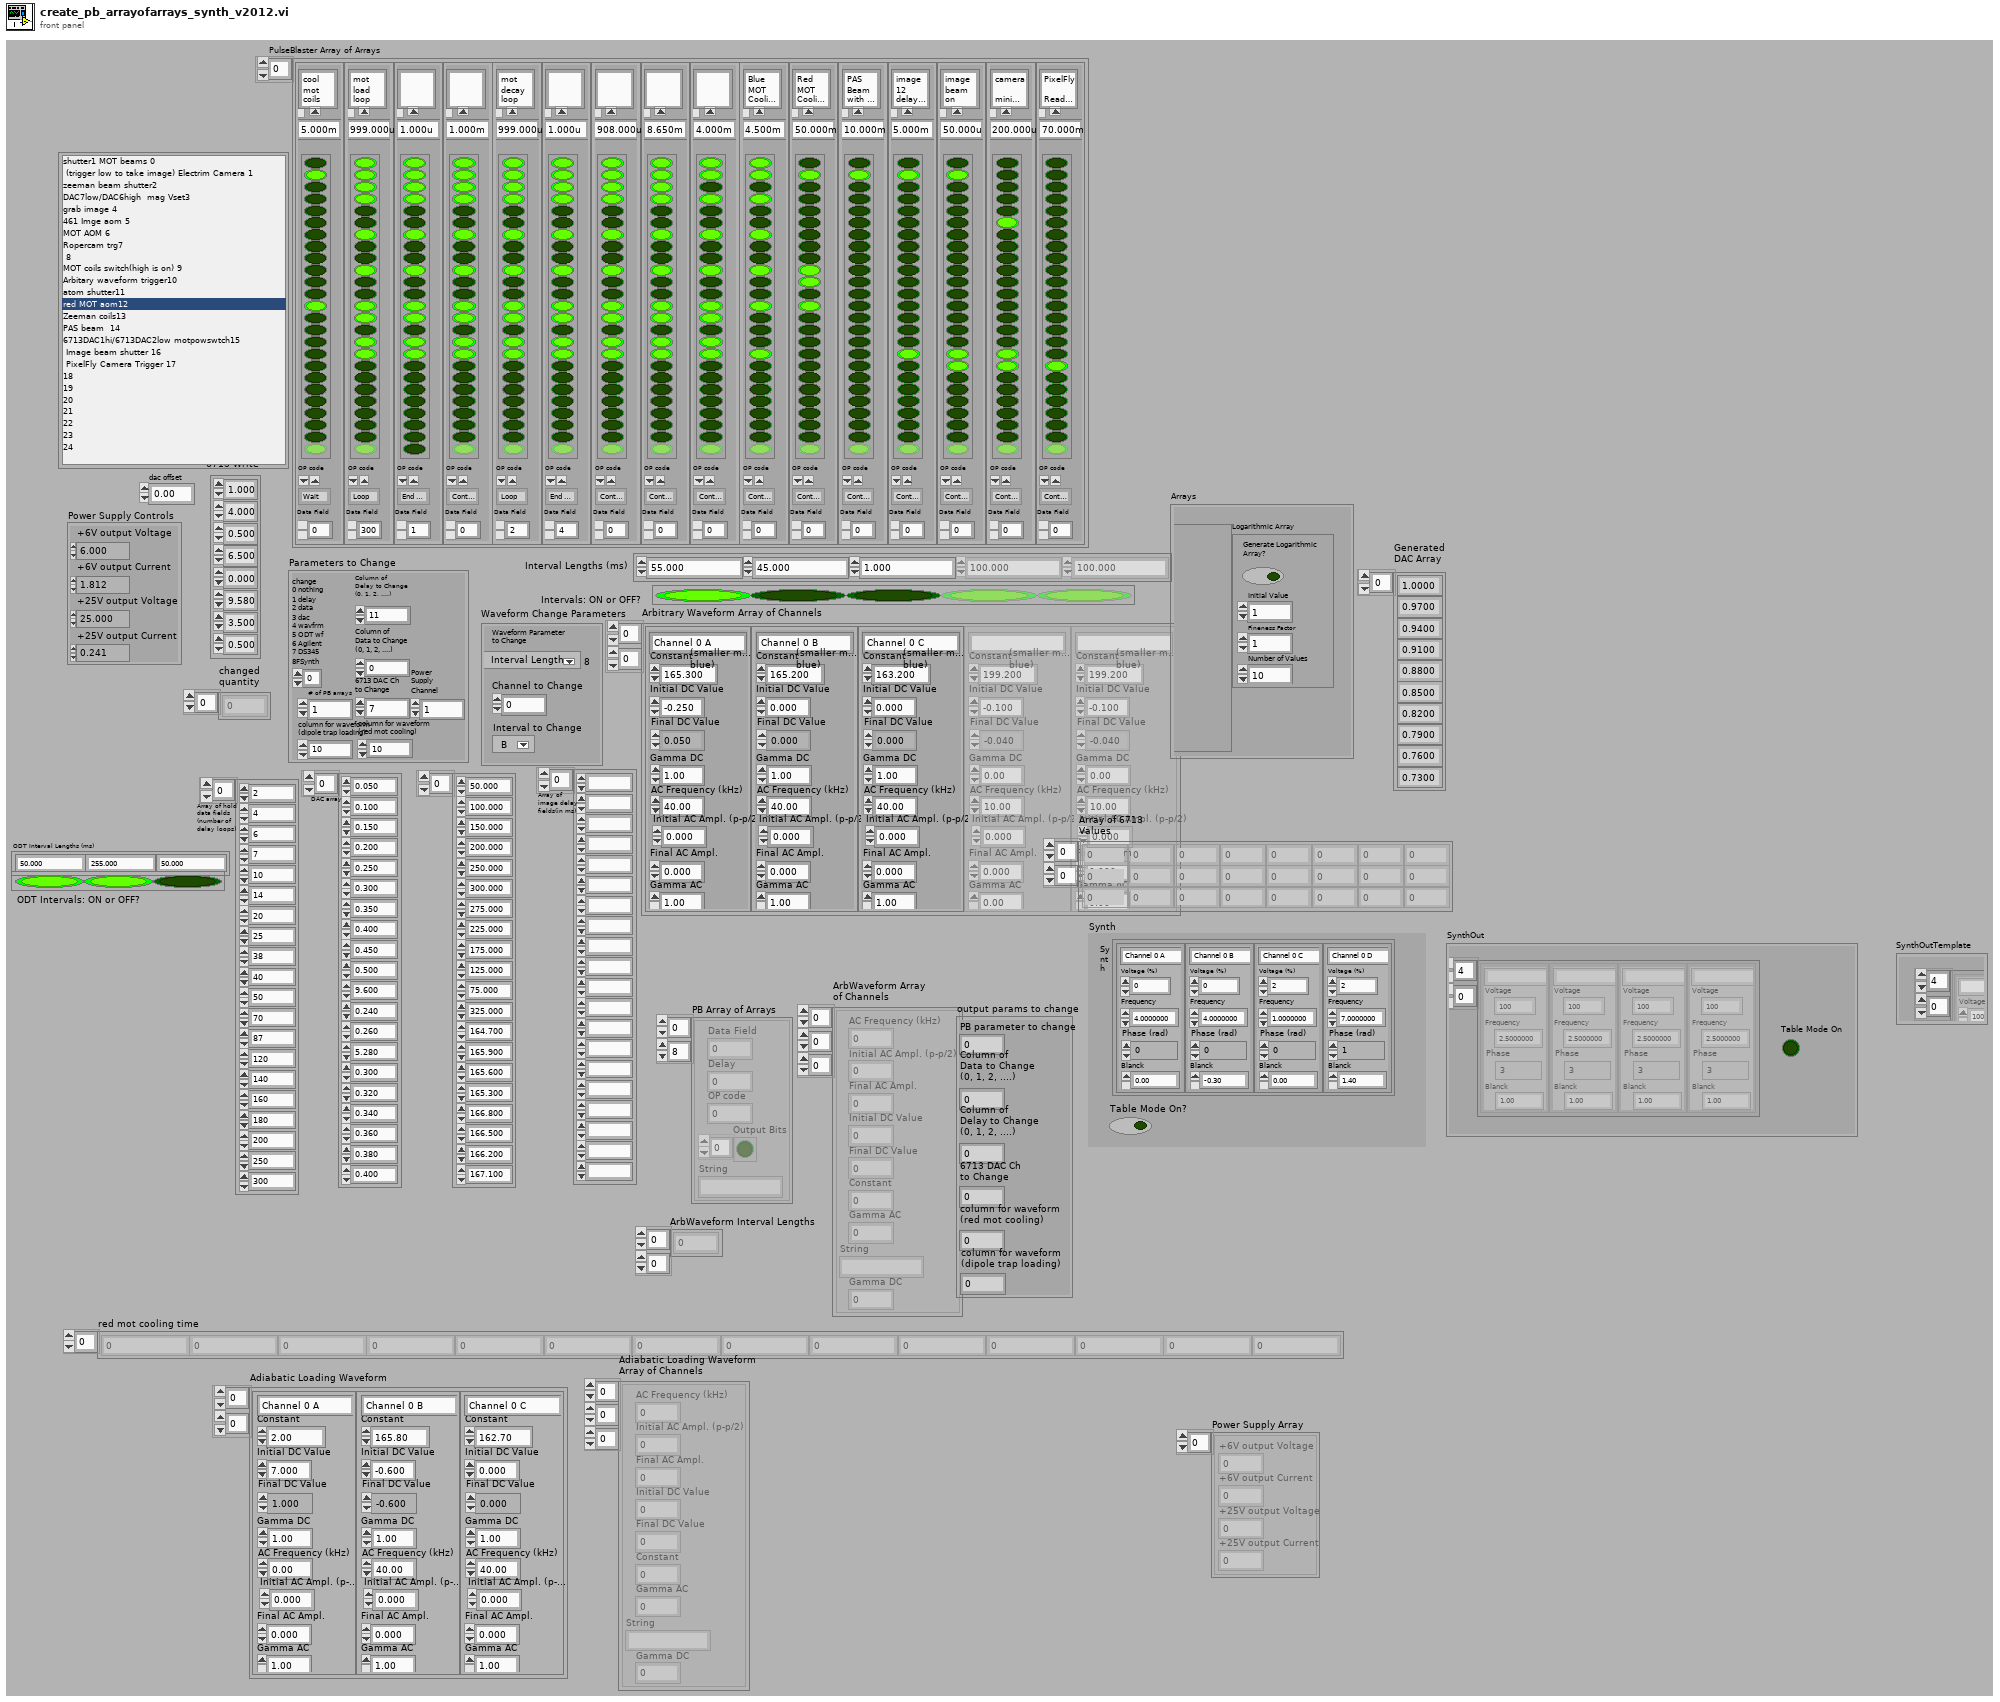
[diagram p1: front panel]
types:
  T1 = cluster{"Table Mode On":bool, "SynthesizerArrayofArrays":cluster{"AC Frequency (kHz)":dbl, " Initial AC Ampl. (p-p/2)":dbl, "Final AC Ampl.":dbl, "Frequency":dbl, "Phase":dbl, "Voltage":dbl, "Gamma AC":dbl, "String":string, "Blanck":dbl}[][]}
  T2 = cluster{"Logarithmic Array":cluster{"Initial Value":i32, "Fineness Factor":i32, "Number of Values":i32, "Generate Logarithmic\nArray?":bool}, "Generated Array":cluster{"Step Size":dbl, "Use generated\nDAC array values?":bool, "Number of DAC Array\nValues to Generate":i32, "Initial Value for DAC":dbl[]}}
  T3 = cluster{"Table Mode On?":bool, "Synth":cluster{"AC Frequency (kHz)":dbl, " Initial AC Ampl. (p-p/2)":dbl, "Final AC Ampl.":dbl, "Frequency":dbl, "Phase (rad)":dbl, "Voltage (%)":dbl, "Gamma AC":dbl, "String":string, "Blanck":dbl}[]}
  T4 = cluster{"+6V output Voltage":dbl, "+6V output Current":dbl, "+25V output Voltage":dbl, "+25V output Current":dbl}[]
  T5 = cluster{"+6V output Voltage":dbl, "+6V output Current":dbl, "+25V output Voltage":dbl, "+25V output Current":dbl}
  T6 = cluster{"AC Frequency (kHz)":dbl, "Initial AC Ampl. (p-p/2)":dbl, "Final AC Ampl.":dbl, "Initial DC Value":dbl, "Final DC Value":dbl, "Constant":dbl, "Gamma AC":dbl, "String":string, "Gamma DC":dbl}[][][]
  T7 = cluster{"AC Frequency (kHz)":dbl, " Initial AC Ampl. (p-p/2)":dbl, "Final AC Ampl.":dbl, "Initial DC Value":dbl, "Final DC Value":dbl, "Constant":dbl, "Gamma AC":dbl, "String":string, "Gamma DC":dbl}[][]
  T8 = cluster{"Channel to Change":i8, "Interval to Change":i8, "Waveform Parameter\nto Change":u16}
  T9 = cluster{"PB parameter to change":i8, "Column of\nData to Change\n(0, 1, 2, ....)":i32, "Column of\nDelay to Change\n(0, 1, 2, ....)":i32, "6713 DAC Ch\nto Change":i32, "column for waveform\n(red mot cooling)":i32, "column for waveform\n(dipole trap loading)":i32}
  T10 = cluster{"PB parameter to change":i8, "Column of\nData to Change\n(0, 1, 2, ....)":i32, "Column of\nDelay to Change\n(0, 1, 2, ....)":i32, "6713 DAC Ch\nto Change":i32, "column for waveform\n(red mot cooling)":i32, "# of PB arrays":i32, "column for waveform\n(dipole trap loading)":i32, "Power\nSupply\nChannel":i32}
  T11 = cluster{"Data Field":u32, "Delay":dbl, "OP code":u8, "Output Bits":bool[], "String":string}[][]
  T12 = cluster{"Data Field":u32, "Delay":dbl, "OP code":u8, "Output Bits":bool[], "String":string}[]
  T13 = cluster{"Initial Value":i32, "Fineness Factor":i32, "Number of Values":i32, "Generate Logarithmic\nArray?":bool}
  T14 = cluster{"Step Size":dbl, "Use generated\nDAC array values?":bool, "Number of DAC Array\nValues to Generate":i32, "Initial Value for DAC":dbl[]}
  T15 = cluster{"AC Frequency (kHz)":dbl, " Initial AC Ampl. (p-p/2)":dbl, "Final AC Ampl.":dbl, "Frequency":dbl, "Phase (rad)":dbl, "Voltage (%)":dbl, "Gamma AC":dbl, "String":string, "Blanck":dbl}[]
  T16 = cluster{"Data Field":u32, "Delay":dbl, "OP code":u8, "Output Bits":bool[], "String":string}
  T17 = cluster{"AC Frequency (kHz)":dbl, " Initial AC Ampl. (p-p/2)":dbl, "Final AC Ampl.":dbl, "Initial DC Value":dbl, "Final DC Value":dbl, "Constant":dbl, "Gamma AC":dbl, "String":string, "Gamma DC":dbl}
  T18 = cluster{"AC Frequency (kHz)":dbl, " Initial AC Ampl. (p-p/2)":dbl, "Final AC Ampl.":dbl, "Frequency":dbl, "Phase (rad)":dbl, "Voltage (%)":dbl, "Gamma AC":dbl, "String":string, "Blanck":dbl}
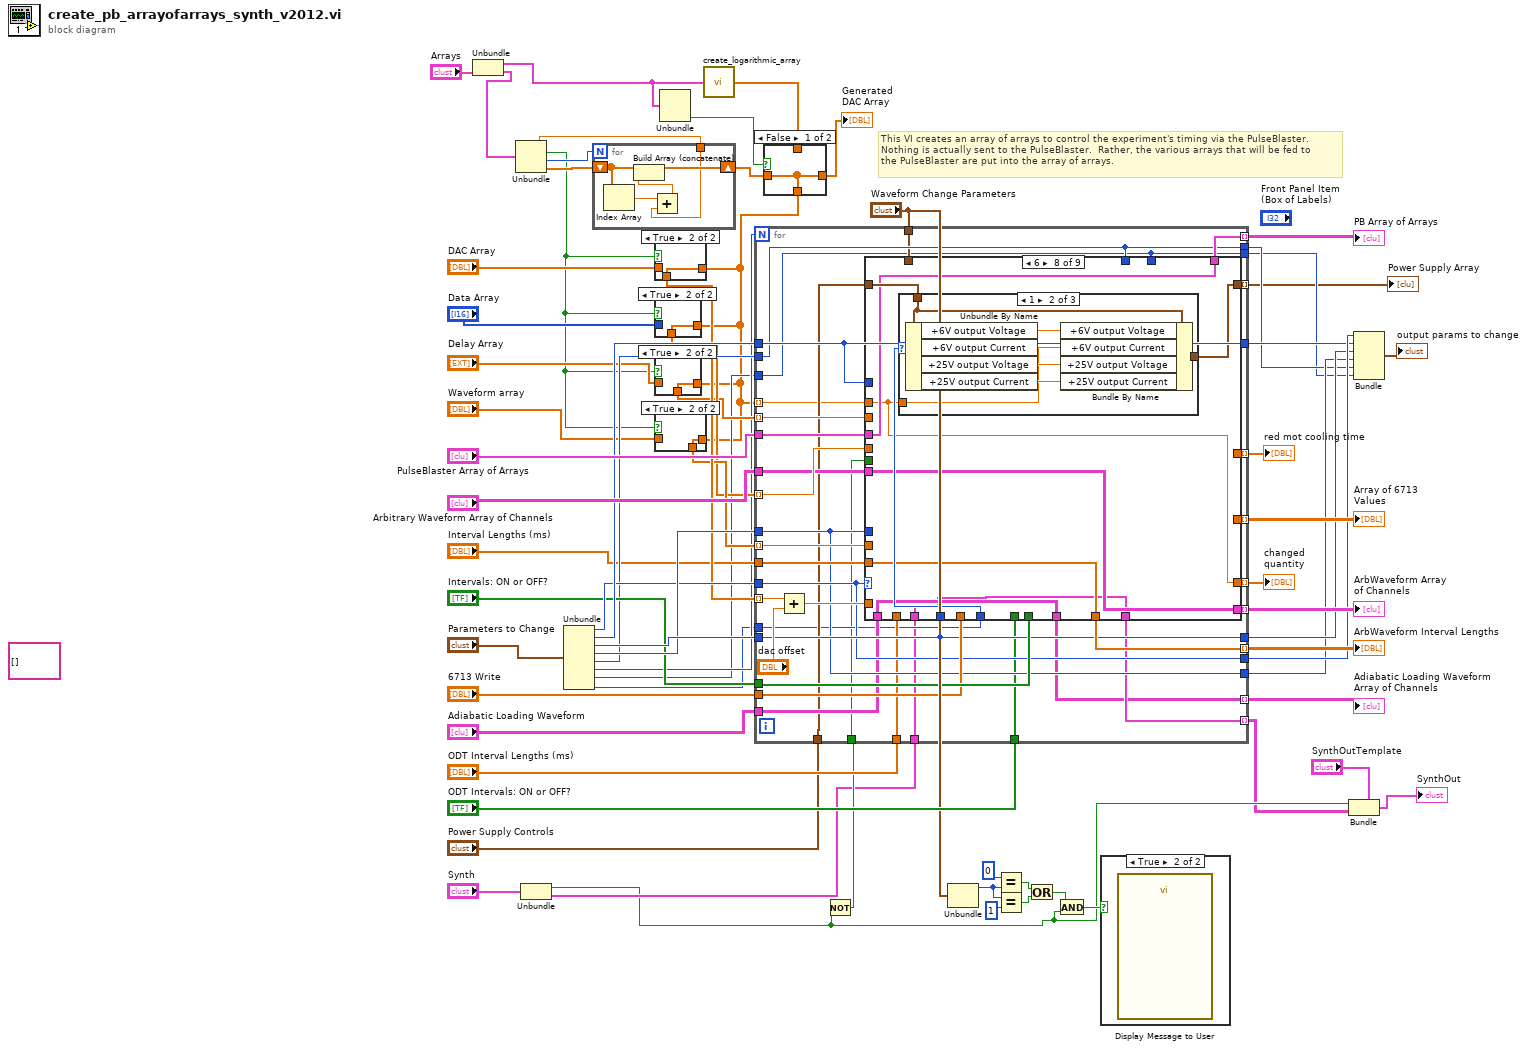
[diagram p0: block diagram]
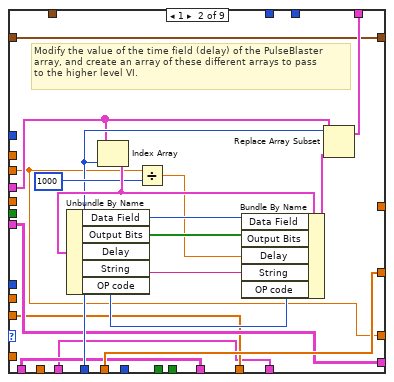
[diagram p9: hidden frame]
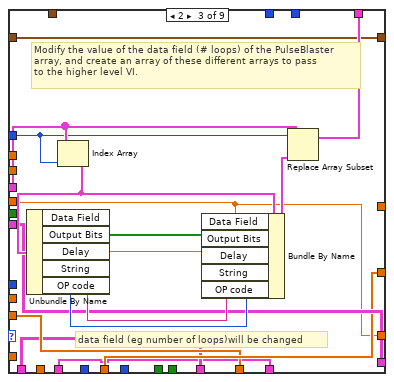
[diagram p10: hidden frame]
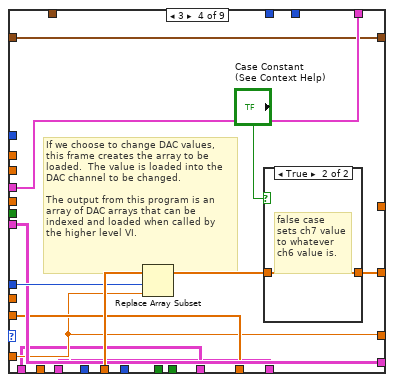
[diagram p11: hidden frame]
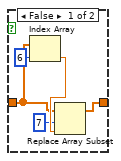
[diagram p12: hidden frame]
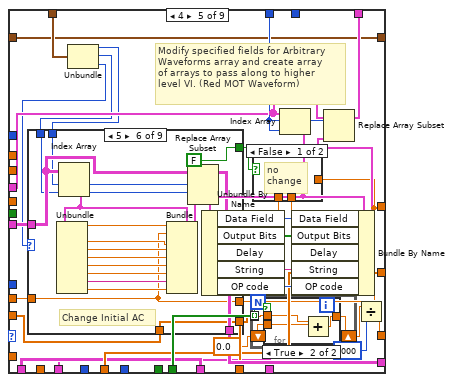
[diagram p13: hidden frame]
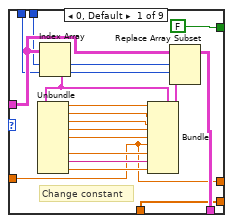
[diagram p16: hidden frame]
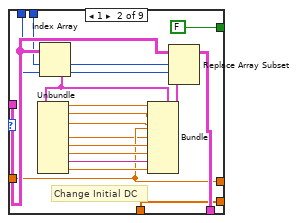
[diagram p17: hidden frame]
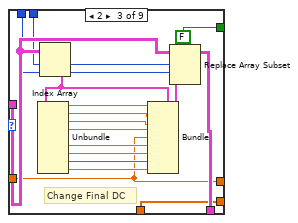
[diagram p18: hidden frame]
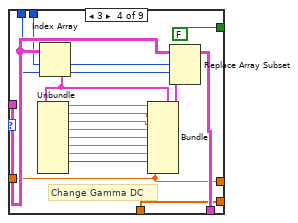
[diagram p19: hidden frame]
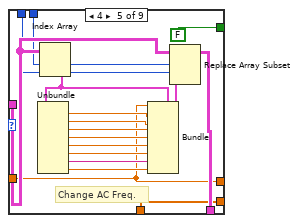
[diagram p20: hidden frame]
diagram:
  (unwired) string[][] [] ("Results")
  # "This VI creates an array of arrays to control the experiment's timing via the PulseBlaster.\nNothing is actually sent to the PulseBlaster.  Rather, the various arrays that will be fed to\nthe PulseBlaster are put into the array of arrays."
  n1 = Unbundle("Arrays") -> ("Logarithmic Array"=w6:T13, "Generated Array"=w5:T14)
  n2 = Unbundle(w5) -> ("Step Size"=w44:dbl, "Use generated\nDAC array values?"=w34:bool, "Number of DAC Array\nValues to Generate"=w45:i32, "Initial Value for DAC"=w46:dbl[])
  n3 = Unbundle("Synth") -> ("Table Mode On?"=w3:bool, "Synth"=w8:T15)
  n4 = Unbundle("Parameters to Change") -> ("PB parameter to change"=w58:i8, "Column of\nData to Change\n(0, 1, 2, ....)"=w59:i32, "Column of\nDelay to Change\n(0, 1, 2, ....)"=w61:i32, "6713 DAC Ch\nto Change"=w60:i32, "column for waveform\n(red mot cooling)"=w49:i32, "# of PB arrays"=w33:i32, "column for waveform\n(dipole trap loading)"=w28:i32, "Power\nSupply\nChannel"=w24:i32)
  n5 = for {
    N: w45 -> [_]
    shift-right: [w74] -> w21
    shift-left: w46 -> [w73]
    tunnel: w44 -> [w69]
    i -> [w72]
    n6 = Index Array(array=w73, index=w72) -> (element=w71:dbl)
    n7 = Add(x=w71, y=w69) -> (x+y=w70:dbl)
    n8 = Build Array (concatenate)(w73, w70) -> (w74:dbl[])
  }
  n9 = Unbundle(w6) -> ("Generate Logarithmic\nArray?"=w22:bool)  [unwired: 3 out]
  n10 = call "create_logarithmic_array.vi"("Logarithmic Array"=w6) -> ("Generated Log Array"=w20:dbl[])
  n11 = case shown="False" w22 {
    tunnel: [w75 w76] -> w23
    tunnel: w21 -> [w75 _]
    tunnel: w20 -> [_ w76]
    tunnel: [w75 w76] -> w19
    frame False {
    }
    frame True {
    }
  }
  "Generated\nDAC Array" <- w23
  n12 = case shown="True" w34 {
    tunnel: w19 -> [_ w78]
    tunnel: "DAC Array" -> [w77 _]
    tunnel: [w77 w78] -> w57
    frame False {
    }
    frame True {
    }
  }
  n13 = case shown="True" w34 {
    tunnel: w19 -> [_ w80]
    tunnel: "Data Array" -> [w79 _]
    tunnel: [w79 w80] -> w37
    frame False {
    }
    frame True {
    }
  }
  n14 = case shown="True" w34 {
    tunnel: w19 -> [_ w82]
    tunnel: "Delay Array" -> [w81 _]
    tunnel: [w81 w82] -> w35
    frame False {
    }
    frame True {
    }
  }
  n15 = case shown="True" w34 {
    tunnel: w19 -> [_ w84]
    tunnel: "Waveform array" -> [w83 _]
    tunnel: [w83 w84] -> w40
    frame False {
    }
    frame True {
    }
  }
  n16 = Not(x=w3) -> (.not. x?=w10:bool)
  n17 = for {
    N: w33 -> [_]
    tunnel: w35 -> [w119] mode=indexing
    tunnel: [w118] -> w50 mode=indexing
    tunnel: [w101] -> w53
    tunnel: w37 -> [w117] mode=indexing
    tunnel: w57 -> [w115] mode=indexing
    tunnel: [w113] -> w68 mode=indexing
    tunnel: w40 -> [w112] mode=indexing
    tunnel: "Intervals: ON or OFF?" -> [w111]
    tunnel: [w110] -> w67 mode=indexing
    tunnel: [w109] -> w66 mode=indexing
    tunnel: "PulseBlaster Array of Arrays" -> [w108]
    tunnel: "Arbitrary Waveform Array of Channels" -> [w107]
    tunnel: w61 -> [w104]
    tunnel: w60 -> [w102]
    tunnel: w59 -> [w101]
    tunnel: w58 -> [w103]
    tunnel: "6713 Write" -> [w106]
    tunnel: "Interval Lengths (ms)" -> [w105]
    tunnel: [w104] -> w52
    tunnel: [w103] -> w54
    tunnel: [w102] -> w51
    tunnel: w49 -> [w100]
    tunnel: [w100] -> w48
    tunnel: [w99] -> w43 mode=indexing
    tunnel: [w98] -> w39 mode=indexing
    tunnel: "Adiabatic Loading Waveform" -> [w97]
    tunnel: "Waveform Change Parameters" -> [w96]
    tunnel: [w86] -> w31 mode=indexing
    tunnel: "ODT Intervals: ON or OFF?" -> [w95]
    tunnel: "ODT Interval Lengths (ms)" -> [w94]
    tunnel: w28 -> [w93]
    tunnel: [w93] -> w27
    tunnel: "Power Supply Controls" -> [w92]
    tunnel: [w91] -> w25 mode=indexing
    tunnel: w24 -> [w90]
    tunnel: w19 -> [w89] mode=indexing
    tunnel: w8 -> [w88]
    tunnel: [w87] -> w2 mode=indexing
    tunnel: w10 -> [w85]
    n18 = Add(x=w115, y="dac offset") -> (x+y=w114:dbl)
    n19 = case shown="6" w103 {
      tunnel: w119 -> [_ w130 _ _ _ _ _ _ _]
      tunnel: w108 -> [w126 w134 w156 w172 w189 w378 w562 w694 w716]
      tunnel: w104 -> [_ w137 _ _ _ _ _ _ _]
      tunnel: [w126 w136 w153 w172 w204 w388 w572 w694 w716] -> w118
      tunnel: w117 -> [_ _ w148 _ _ _ _ _ _]
      tunnel: w106 -> [w125 w135 w151 w171 w191 w379 w563 _ _]
      tunnel: w114 -> [_ _ _ w167 _ _ _ _ _]
      tunnel: [w125 w135 w151 w162 w191 w379 w563 _ _] -> w113
      tunnel: w102 -> [_ _ _ w170 _ _ _ _ _]
      tunnel: w100 -> [_ _ _ _ w203 _ _ _ _]
      tunnel: w107 -> [w124 w133 w152 w169 w200 w368 w556 w692 w715]
      tunnel: w112 -> [_ _ _ _ w199 w385 w569 _ _]
      tunnel: [w124 w133 w152 w169 w198 w368 w556 w692 w715] -> w110
      tunnel: w111 -> [_ _ _ _ w197 _ _ _ _]
      tunnel: [w123 w132 w150 w168 w195 w363 w551 w691 w713] -> w109
      tunnel: w105 -> [w123 w132 w150 w168 w190 w363 w551 w691 w713]
      tunnel: w101 -> [_ _ w149 _ _ _ _ _ _]
      tunnel: [_ w130 w148 w167 w187 w376 w560 w690 w717] -> w99
      tunnel: [_ _ _ _ w181 w372 w558 _ _] -> w98
      tunnel: w97 -> [w122 w129 w147 w166 w182 w371 w549 w693 w712]
      tunnel: w96 -> [_ _ _ _ w183 w370 w557 _ _]
      tunnel: [w122 w129 w147 w166 w182 w369 w549 w693 w712] -> w86
      tunnel: w95 -> [_ _ _ _ _ w367 w555 _ _]
      tunnel: w94 -> [_ _ _ _ _ w366 w554 _ _]
      tunnel: w93 -> [_ _ _ _ _ w365 w553 _ _]
      tunnel: w92 -> [w121 w128 w146 w165 w180 w364 w552 w697 w714]
      tunnel: [w121 w128 w146 w165 w180 w364 w552 w696 w714] -> w91
      tunnel: w90 -> [_ _ _ _ _ _ _ w695 _]
      tunnel: w89 -> [_ _ _ _ _ _ _ w690 w717]
      tunnel: w88 -> [w120 w127 w145 w161 w179 w362 w550 w689 w711]
      tunnel: [w120 w127 w145 w161 w179 w362 w547 w689 w711] -> w87
      tunnel: w85 -> [_ _ _ _ _ _ w546 _ _]
      frame 0, Default {
        # "No arrays modified.\nPass them on as is."
      }
      frame 1 {
        # "Modify the value of the time field (delay) of the PulseBlaster\narray, and create an array of these different arrays to pass\nto the higher level VI."
        n20 = Index Array(array=w134, index=w137) -> (element=w142:T16)
        n21 = Unbundle By Name(w142) -> ("Data Field"=w139:u32, "Output Bits"=w141:bool[], "String"=w144:string, "OP code"=w143:u8)  [unwired: 1 out]
        n22 = Divide(x=w130, y=1000) -> (x/y=w131:ext)
        n23 = Bundle By Name(cluster=w142, "Data Field"=w139, "Output Bits"=w141, "Delay"=w131, "String"=w144, "OP code"=w143) -> (w140:T16)
        n24 = Replace Array Subset(array=w134, new element=w140, index=w137) -> (w136:T12)
      }
      frame 2 {
        # "Modify the value of the data field (# loops) of the PulseBlaster\narray, and create an array of these different arrays to pass\nto the higher level VI."
        # "data field (eg number of loops)will be changed"
        n25 = Index Array(array=w156, index=w149) -> (element=w155:T16)
        n26 = Unbundle By Name(w155) -> ("Output Bits"=w158:bool[], "Delay"=w154:dbl, "String"=w160:string, "OP code"=w159:u8)  [unwired: 1 out]
        n27 = Bundle By Name(cluster=w155, "Data Field"=w148, "Output Bits"=w158, "Delay"=w154, "String"=w160, "OP code"=w159) -> (w157:T16)
        n28 = Replace Array Subset(array=w156, new element=w157, index=w149) -> (w153:T12)
      }
      frame 3 {
        # "If we choose to change DAC values,\nthis frame creates the array to be\nloaded.  The value is loaded into the\nDAC channel to be changed.\n\nThe output from this program is an\narray of DAC arrays that can be\nindexed and loaded when called by\nthe higher level VI."
        n29 = Replace Array Subset(array=w171, new element=w167, index=w170) -> (w163:dbl[])
        n30 = case shown="True" "Case Constant\n(See Context Help)" {
          tunnel: w163 -> [w174 w178]
          tunnel: [w173 w178] -> w162
          frame False {
            n31 = Index Array(array=w174, index=6) -> (element=w176:dbl)
            n32 = Replace Array Subset(array=w174, new element=w176, index=7) -> (w173:dbl[])
          }
          frame True {
            # "false case\nsets ch7 value\nto whatever\nch6 value is."
          }
        }
      }
      frame 4 {
        # "Modify specified fields for Arbitrary\nWaveforms array and create array\nof arrays to pass along to higher\nlevel VI. (Red MOT Waveform)"
        n33 = Unbundle(w183) -> ("Channel to Change"=w186:i8, "Interval to Change"=w185:i8, "Waveform Parameter\nto Change"=w184:u16)
        n34 = case shown="5" w184 {
          tunnel: w200 -> [w227 w245 w261 w278 w295 w312 w329 w346 w361]
          tunnel: w186 -> [w220 w244 w260 w277 w294 w311 w328 w345 _]
          tunnel: w185 -> [w226 w243 w259 w276 w293 w310 w327 w344 w359]
          tunnel: w199 -> [w221 w238 w254 w271 w288 w305 w322 w339 w356]
          tunnel: [w224 w241 w257 w274 w291 w308 w325 w342 w361] -> w198
          tunnel: w190 -> [w223 w240 w256 w273 w290 w307 w324 w340 w360]
          tunnel: [w223 w240 w256 w273 w290 w307 w324 w340 w358] -> w195
          tunnel: [FALSE FALSE FALSE FALSE FALSE FALSE FALSE FALSE TRUE] -> w188
          tunnel: [w221 w238 w254 w271 w288 w305 w322 w339 w356] -> w187
          frame 0, Default {
            # "Change constant"
            n35 = Index Array(array=w227, index (row)=w220, index (col)=w226) -> (element=w236:T17)
            n36 = Unbundle(w236) -> ("AC Frequency (kHz)"=w235:dbl, "Initial AC Ampl. (p-p/2)"=w234:dbl, "Final AC Ampl."=w233:dbl, "Initial DC Value"=w232:dbl, "Final DC Value"=w231:dbl, "Gamma AC"=w230:dbl, "String"=w228:string, "Gamma DC"=w229:dbl)  [unwired: 1 out]
            n37 = Bundle(cluster=w236, "AC Frequency (kHz)"=w235, "Initial AC Ampl. (p-p/2)"=w234, "Final AC Ampl."=w233, "Initial DC Value"=w232, "Final DC Value"=w231, "Constant"=w221, "Gamma AC"=w230, "String"=w228, "Gamma DC"=w229) -> (w225:T17)
            n38 = Replace Array Subset(array=w227, new element=w225, index (row)=w220, index (col)=w226) -> (w224:T7)
          }
          frame 1 {
            # "Change Initial DC"
            n39 = Index Array(array=w245, index (row)=w244, index (col)=w243) -> (element=w253:T17)
            n40 = Unbundle(w253) -> ("AC Frequency (kHz)"=w252:dbl, "Initial AC Ampl. (p-p/2)"=w251:dbl, "Final AC Ampl."=w250:dbl, "Final DC Value"=w237:dbl, "Constant"=w249:dbl, "Gamma AC"=w248:dbl, "String"=w246:string, "Gamma DC"=w247:dbl)  [unwired: 1 out]
            n41 = Bundle(cluster=w253, "AC Frequency (kHz)"=w252, "Initial AC Ampl. (p-p/2)"=w251, "Final AC Ampl."=w250, "Initial DC Value"=w238, "Final DC Value"=w237, "Constant"=w249, "Gamma AC"=w248, "String"=w246, "Gamma DC"=w247) -> (w242:T17)
            n42 = Replace Array Subset(array=w245, new element=w242, index (row)=w244, index (col)=w243) -> (w241:T7)
          }
          frame 2 {
            # "Change Final DC"
            n43 = Index Array(array=w261, index (row)=w260, index (col)=w259) -> (element=w270:T17)
            n44 = Unbundle(w270) -> ("AC Frequency (kHz)"=w269:dbl, "Initial AC Ampl. (p-p/2)"=w268:dbl, "Final AC Ampl."=w267:dbl, "Initial DC Value"=w266:dbl, "Constant"=w265:dbl, "Gamma AC"=w264:dbl, "String"=w262:string, "Gamma DC"=w263:dbl)  [unwired: 1 out]
            n45 = Bundle(cluster=w270, "AC Frequency (kHz)"=w269, "Initial AC Ampl. (p-p/2)"=w268, "Final AC Ampl."=w267, "Initial DC Value"=w266, "Final DC Value"=w254, "Constant"=w265, "Gamma AC"=w264, "String"=w262, "Gamma DC"=w263) -> (w258:T17)
            n46 = Replace Array Subset(array=w261, new element=w258, index (row)=w260, index (col)=w259) -> (w257:T7)
          }
          frame 3 {
            # "Change Gamma DC"
            n47 = Index Array(array=w278, index (row)=w277, index (col)=w276) -> (element=w287:T17)
            n48 = Unbundle(w287) -> ("AC Frequency (kHz)"=w286:dbl, "Initial AC Ampl. (p-p/2)"=w285:dbl, "Final AC Ampl."=w284:dbl, "Initial DC Value"=w283:dbl, "Final DC Value"=w282:dbl, "Constant"=w281:dbl, "Gamma AC"=w280:dbl, "String"=w279:string)  [unwired: 1 out]
            n49 = Bundle(cluster=w287, "AC Frequency (kHz)"=w286, "Initial AC Ampl. (p-p/2)"=w285, "Final AC Ampl."=w284, "Initial DC Value"=w283, "Final DC Value"=w282, "Constant"=w281, "Gamma AC"=w280, "String"=w279, "Gamma DC"=w271) -> (w275:T17)
            n50 = Replace Array Subset(array=w278, new element=w275, index (row)=w277, index (col)=w276) -> (w274:T7)
          }
          frame 4 {
            # "Change AC Freq."
            n51 = Index Array(array=w295, index (row)=w294, index (col)=w293) -> (element=w304:T17)
            n52 = Unbundle(w304) -> ("Initial AC Ampl. (p-p/2)"=w303:dbl, "Final AC Ampl."=w302:dbl, "Initial DC Value"=w301:dbl, "Final DC Value"=w300:dbl, "Constant"=w299:dbl, "Gamma AC"=w298:dbl, "String"=w296:string, "Gamma DC"=w297:dbl)  [unwired: 1 out]
            n53 = Bundle(cluster=w304, "AC Frequency (kHz)"=w288, "Initial AC Ampl. (p-p/2)"=w303, "Final AC Ampl."=w302, "Initial DC Value"=w301, "Final DC Value"=w300, "Constant"=w299, "Gamma AC"=w298, "String"=w296, "Gamma DC"=w297) -> (w292:T17)
            n54 = Replace Array Subset(array=w295, new element=w292, index (row)=w294, index (col)=w293) -> (w291:T7)
          }
          frame 5 {
            # "Change Initial AC"
            n55 = Index Array(array=w312, index (row)=w311, index (col)=w310) -> (element=w321:T17)
            n56 = Unbundle(w321) -> ("AC Frequency (kHz)"=w320:dbl, "Final AC Ampl."=w319:dbl, "Initial DC Value"=w318:dbl, "Final DC Value"=w317:dbl, "Constant"=w316:dbl, "Gamma AC"=w315:dbl, "String"=w313:string, "Gamma DC"=w314:dbl)  [unwired: 1 out]
            n57 = Bundle(cluster=w321, "AC Frequency (kHz)"=w320, "Initial AC Ampl. (p-p/2)"=w305, "Final AC Ampl."=w319, "Initial DC Value"=w318, "Final DC Value"=w317, "Constant"=w316, "Gamma AC"=w315, "String"=w313, "Gamma DC"=w314) -> (w309:T17)
            n58 = Replace Array Subset(array=w312, new element=w309, index (row)=w311, index (col)=w310) -> (w308:T7)
          }
          frame 6 {
            # "Change Final AC"
            n59 = Index Array(array=w329, index (row)=w328, index (col)=w327) -> (element=w338:T17)
            n60 = Unbundle(w338) -> ("AC Frequency (kHz)"=w337:dbl, "Initial AC Ampl. (p-p/2)"=w336:dbl, "Initial DC Value"=w335:dbl, "Final DC Value"=w334:dbl, "Constant"=w333:dbl, "Gamma AC"=w332:dbl, "String"=w330:string, "Gamma DC"=w331:dbl)  [unwired: 1 out]
            n61 = Bundle(cluster=w338, "AC Frequency (kHz)"=w337, "Initial AC Ampl. (p-p/2)"=w336, "Final AC Ampl."=w322, "Initial DC Value"=w335, "Final DC Value"=w334, "Constant"=w333, "Gamma AC"=w332, "String"=w330, "Gamma DC"=w331) -> (w326:T17)
            n62 = Replace Array Subset(array=w329, new element=w326, index (row)=w328, index (col)=w327) -> (w325:T7)
          }
          frame 7 {
            # "Change Gamma AC"
            n63 = Index Array(array=w346, index (row)=w345, index (col)=w344) -> (element=w355:T17)
            n64 = Unbundle(w355) -> ("AC Frequency (kHz)"=w354:dbl, "Initial AC Ampl. (p-p/2)"=w353:dbl, "Final AC Ampl."=w352:dbl, "Initial DC Value"=w351:dbl, "Final DC Value"=w350:dbl, "Constant"=w349:dbl, "String"=w347:string, "Gamma DC"=w348:dbl)  [unwired: 1 out]
            n65 = Bundle(cluster=w355, "AC Frequency (kHz)"=w354, "Initial AC Ampl. (p-p/2)"=w353, "Final AC Ampl."=w352, "Initial DC Value"=w351, "Final DC Value"=w350, "Constant"=w349, "Gamma AC"=w339, "String"=w347, "Gamma DC"=w348) -> (w343:T17)
            n66 = Replace Array Subset(array=w346, new element=w343, index (row)=w345, index (col)=w344) -> (w342:T7)
          }
          frame 8 {
            # "Change Time Interval"
            n67 = Replace Array Subset(array=w360, new element=w356, index=w359) -> (w358:dbl[])
          }
        }
        n68 = for {
          tunnel: w195 -> [w213] mode=indexing
          tunnel: w197 -> [w215] mode=indexing
          shift-right: [w212] -> w196
          shift-left: 0.0 -> [w214]
          n69 = case shown="True" w215 {
            tunnel: w214 -> [w216 w219]
            tunnel: w213 -> [_ w218]
            tunnel: [w216 w217] -> w212
            frame False {
              # "zero s"
            }
            frame True {
              n70 = Add(x=w218, y=w219) -> (x+y=w217:dbl)
            }
          }
        }
        n71 = Index Array(array=w189, index=w203) -> (element=w209:T16)
        n72 = Unbundle By Name(w209) -> ("Data Field"=w206:u32, "Output Bits"=w208:bool[], "Delay"=w193:dbl, "String"=w202:string, "OP code"=w201:u8)
        n73 = Divide(x=w196, y=1000) -> (x/y=w181:dbl)
        n74 = case shown="False" w188 {
          tunnel: w193 -> [w210 _]
          tunnel: [w210 w211] -> w192
          tunnel: w181 -> [_ w211]
          frame False {
            # "no \nchange"
          }
          frame True {
            # "match \nintervals"
          }
        }
        n75 = Bundle By Name(cluster=w209, "Data Field"=w206, "Output Bits"=w208, "Delay"=w192, "String"=w202, "OP code"=w201) -> (w207:T16)
        n76 = Replace Array Subset(array=w189, new element=w207, index=w203) -> (w204:T12)
      }
      frame 5 {
        # "Modify specified fields for Arbitrary\nWaveforms array and create array\nof arrays to pass along to higher\nlevel VI. (ODT Loading Waveform)"
        n77 = Unbundle(w370) -> ("Channel to Change"=w375:i8, "Interval to Change"=w374:i8, "Waveform Parameter\nto Change"=w373:u16)
        n78 = case shown="7" w373 {
          tunnel: w371 -> [w411 w428 w445 w462 w472 w496 w513 w530 w545]
          tunnel: w375 -> [w404 w427 w444 w461 w479 w495 w512 w529 _]
          tunnel: w374 -> [w410 w426 w443 w460 w478 w494 w511 w528 w543]
          tunnel: w385 -> [w405 w421 w438 w455 w473 w489 w506 w523 w540]
          tunnel: [w408 w424 w441 w458 w476 w492 w509 w526 w545] -> w369
          tunnel: w366 -> [w407 w423 w440 w457 w475 w491 w508 w524 w544]
          tunnel: [w407 w423 w440 w457 w475 w491 w508 w524 w542] -> w383
          tunnel: [FALSE FALSE FALSE FALSE FALSE FALSE FALSE TRUE TRUE] -> w377
          tunnel: [w405 w421 w438 w455 w473 w489 w506 w523 w540] -> w376
          frame 0, Default {
            # "Change constant"
            n79 = Index Array(array=w411, index (row)=w404, index (col)=w410) -> (element=w420:T17)
            n80 = Unbundle(w420) -> ("AC Frequency (kHz)"=w419:dbl, "Initial AC Ampl. (p-p/2)"=w418:dbl, "Final AC Ampl."=w417:dbl, "Initial DC Value"=w416:dbl, "Final DC Value"=w415:dbl, "Gamma AC"=w414:dbl, "String"=w412:string, "Gamma DC"=w413:dbl)  [unwired: 1 out]
            n81 = Bundle(cluster=w420, "AC Frequency (kHz)"=w419, "Initial AC Ampl. (p-p/2)"=w418, "Final AC Ampl."=w417, "Initial DC Value"=w416, "Final DC Value"=w415, "Constant"=w405, "Gamma AC"=w414, "String"=w412, "Gamma DC"=w413) -> (w409:T17)
            n82 = Replace Array Subset(array=w411, new element=w409, index (row)=w404, index (col)=w410) -> (w408:T7)
          }
          frame 1 {
            # "Change Initial DC"
            n83 = Index Array(array=w428, index (row)=w427, index (col)=w426) -> (element=w437:T17)
            n84 = Unbundle(w437) -> ("AC Frequency (kHz)"=w436:dbl, "Initial AC Ampl. (p-p/2)"=w435:dbl, "Final AC Ampl."=w434:dbl, "Final DC Value"=w433:dbl, "Constant"=w432:dbl, "Gamma AC"=w431:dbl, "String"=w429:string, "Gamma DC"=w430:dbl)  [unwired: 1 out]
            n85 = Bundle(cluster=w437, "AC Frequency (kHz)"=w436, "Initial AC Ampl. (p-p/2)"=w435, "Final AC Ampl."=w434, "Initial DC Value"=w421, "Final DC Value"=w433, "Constant"=w432, "Gamma AC"=w431, "String"=w429, "Gamma DC"=w430) -> (w425:T17)
            n86 = Replace Array Subset(array=w428, new element=w425, index (row)=w427, index (col)=w426) -> (w424:T7)
          }
          frame 2 {
            # "Change Final DC"
            n87 = Index Array(array=w445, index (row)=w444, index (col)=w443) -> (element=w454:T17)
            n88 = Unbundle(w454) -> ("AC Frequency (kHz)"=w453:dbl, "Initial AC Ampl. (p-p/2)"=w452:dbl, "Final AC Ampl."=w451:dbl, "Initial DC Value"=w450:dbl, "Constant"=w449:dbl, "Gamma AC"=w448:dbl, "String"=w446:string, "Gamma DC"=w447:dbl)  [unwired: 1 out]
            n89 = Bundle(cluster=w454, "AC Frequency (kHz)"=w453, "Initial AC Ampl. (p-p/2)"=w452, "Final AC Ampl."=w451, "Initial DC Value"=w450, "Final DC Value"=w438, "Constant"=w449, "Gamma AC"=w448, "String"=w446, "Gamma DC"=w447) -> (w442:T17)
            n90 = Replace Array Subset(array=w445, new element=w442, index (row)=w444, index (col)=w443) -> (w441:T7)
          }
          frame 3 {
            # "Change Gamma DC"
            n91 = Index Array(array=w462, index (row)=w461, index (col)=w460) -> (element=w471:T17)
            n92 = Unbundle(w471) -> ("AC Frequency (kHz)"=w470:dbl, "Initial AC Ampl. (p-p/2)"=w469:dbl, "Final AC Ampl."=w468:dbl, "Initial DC Value"=w467:dbl, "Final DC Value"=w466:dbl, "Constant"=w465:dbl, "Gamma AC"=w464:dbl, "String"=w463:string)  [unwired: 1 out]
            n93 = Bundle(cluster=w471, "AC Frequency (kHz)"=w470, "Initial AC Ampl. (p-p/2)"=w469, "Final AC Ampl."=w468, "Initial DC Value"=w467, "Final DC Value"=w466, "Constant"=w465, "Gamma AC"=w464, "String"=w463, "Gamma DC"=w455) -> (w459:T17)
            n94 = Replace Array Subset(array=w462, new element=w459, index (row)=w461, index (col)=w460) -> (w458:T7)
          }
          frame 4 {
            # "Change AC Freq."
            n95 = Index Array(array=w472, index (row)=w479, index (col)=w478) -> (element=w488:T17)
            n96 = Unbundle(w488) -> ("Initial AC Ampl. (p-p/2)"=w487:dbl, "Final AC Ampl."=w486:dbl, "Initial DC Value"=w485:dbl, "Final DC Value"=w484:dbl, "Constant"=w483:dbl, "Gamma AC"=w482:dbl, "String"=w480:string, "Gamma DC"=w481:dbl)  [unwired: 1 out]
            n97 = Bundle(cluster=w488, "AC Frequency (kHz)"=w473, "Initial AC Ampl. (p-p/2)"=w487, "Final AC Ampl."=w486, "Initial DC Value"=w485, "Final DC Value"=w484, "Constant"=w483, "Gamma AC"=w482, "String"=w480, "Gamma DC"=w481) -> (w477:T17)
            n98 = Replace Array Subset(array=w472, new element=w477, index (row)=w479, index (col)=w478) -> (w476:T7)
          }
          frame 5 {
            # "Change Initial AC"
            n99 = Index Array(array=w496, index (row)=w495, index (col)=w494) -> (element=w505:T17)
            n100 = Unbundle(w505) -> ("AC Frequency (kHz)"=w504:dbl, "Final AC Ampl."=w503:dbl, "Initial DC Value"=w502:dbl, "Final DC Value"=w501:dbl, "Constant"=w500:dbl, "Gamma AC"=w499:dbl, "String"=w497:string, "Gamma DC"=w498:dbl)  [unwired: 1 out]
            n101 = Bundle(cluster=w505, "AC Frequency (kHz)"=w504, "Initial AC Ampl. (p-p/2)"=w489, "Final AC Ampl."=w503, "Initial DC Value"=w502, "Final DC Value"=w501, "Constant"=w500, "Gamma AC"=w499, "String"=w497, "Gamma DC"=w498) -> (w493:T17)
            n102 = Replace Array Subset(array=w496, new element=w493, index (row)=w495, index (col)=w494) -> (w492:T7)
          }
          frame 6 {
            # "Change Final AC"
            n103 = Index Array(array=w513, index (row)=w512, index (col)=w511) -> (element=w522:T17)
            n104 = Unbundle(w522) -> ("AC Frequency (kHz)"=w521:dbl, "Initial AC Ampl. (p-p/2)"=w520:dbl, "Initial DC Value"=w519:dbl, "Final DC Value"=w518:dbl, "Constant"=w517:dbl, "Gamma AC"=w516:dbl, "String"=w514:string, "Gamma DC"=w515:dbl)  [unwired: 1 out]
            n105 = Bundle(cluster=w522, "AC Frequency (kHz)"=w521, "Initial AC Ampl. (p-p/2)"=w520, "Final AC Ampl."=w506, "Initial DC Value"=w519, "Final DC Value"=w518, "Constant"=w517, "Gamma AC"=w516, "String"=w514, "Gamma DC"=w515) -> (w510:T17)
            n106 = Replace Array Subset(array=w513, new element=w510, index (row)=w512, index (col)=w511) -> (w509:T7)
          }
          frame 7 {
            # "Change Gamma AC"
            n107 = Index Array(array=w530, index (row)=w529, index (col)=w528) -> (element=w539:T17)
            n108 = Unbundle(w539) -> ("AC Frequency (kHz)"=w538:dbl, "Initial AC Ampl. (p-p/2)"=w537:dbl, "Final AC Ampl."=w536:dbl, "Initial DC Value"=w535:dbl, "Final DC Value"=w534:dbl, "Constant"=w533:dbl, "String"=w531:string, "Gamma DC"=w532:dbl)  [unwired: 1 out]
            n109 = Bundle(cluster=w539, "AC Frequency (kHz)"=w538, "Initial AC Ampl. (p-p/2)"=w537, "Final AC Ampl."=w536, "Initial DC Value"=w535, "Final DC Value"=w534, "Constant"=w533, "Gamma AC"=w523, "String"=w531, "Gamma DC"=w532) -> (w527:T17)
            n110 = Replace Array Subset(array=w530, new element=w527, index (row)=w529, index (col)=w528) -> (w526:T7)
          }
          frame 8 {
            # "Change Time Interval"
            n111 = Replace Array Subset(array=w544, new element=w540, index=w543) -> (w542:dbl[])
          }
        }
        n112 = for {
          tunnel: w383 -> [w397] mode=indexing
          tunnel: w367 -> [w399] mode=indexing
          shift-right: [w396] -> w384
          shift-left: 0.0 -> [w398]
          n113 = case shown="False" w399 {
            tunnel: w398 -> [w400 w403]
            tunnel: w397 -> [_ w402]
            tunnel: [w400 w401] -> w396
            frame False {
              # "zero s"
            }
            frame True {
              n114 = Add(x=w402, y=w403) -> (x+y=w401:dbl)
            }
          }
        }
        n115 = Index Array(array=w378, index=w365) -> (element=w393:T16)
        n116 = Unbundle By Name(w393) -> ("Data Field"=w390:u32, "Output Bits"=w392:bool[], "Delay"=w381:dbl, "String"=w387:string, "OP code"=w386:u8)
        n117 = Divide(x=w384, y=1000) -> (x/y=w372:dbl)
        n118 = case shown="False" w377 {
          tunnel: w381 -> [w394 _]
          tunnel: [w394 w395] -> w380
          tunnel: w372 -> [_ w395]
          frame False {
            # "no \nchange"
          }
          frame True {
            # "match \nintevals"
          }
        }
        n119 = Bundle By Name(cluster=w393, "Data Field"=w390, "Output Bits"=w392, "Delay"=w380, "String"=w387, "OP code"=w386) -> (w391:T16)
        n120 = Replace Array Subset(array=w378, new element=w391, index=w365) -> (w388:T12)
      }
      frame 9 {
        # "Modify specified fields for Arbitrary\nWaveforms array and create array\nof arrays to pass along to higher\nlevel VI. (ODT Loading Waveform)"
        n121 = Unbundle(w557) -> ("Channel to Change"=w548:i8, "Interval to Change"=w559:i8)  [unwired: 1 out]
        n122 = case shown="0, Default" w548 {
          tunnel: w548 -> [w592 w615 w645 w659 w676]
          tunnel: w559 -> [_ _ _ _ _]
          tunnel: w569 -> [w589 w618 w641 w657 w673]
          tunnel: w554 -> [w594 w620 w648 w664 w681]
          tunnel: [w594 w620 w648 w664 w681] -> w567
          tunnel: [FALSE FALSE FALSE FALSE TRUE] -> w561
          tunnel: [w588 w617 w641 w657 w673] -> w560
          tunnel: w550 -> [w593 w619 w643 w662 w679]
          tunnel: [w591 w616 w638 w655 w672] -> w547
          tunnel: w546 -> [w590 w614 _ _ _]
          frame 0, Default {
            n123 = case shown="False" w590 {
              tunnel: w593 -> [w597 w601]
              tunnel: w592 -> [_ w600]
              tunnel: [w597 w599] -> w591
              tunnel: w589 -> [w596 w598]
              tunnel: [w596 w598] -> w588
              frame False {
              }
              frame True {
                n124 = Index Array(array=w601, index #1=w600, index #2=1) -> (element #1=w603:T18)  [unwired: 1 out]
                n125 = Unbundle(w603) -> ("AC Frequency (kHz)"=w612:dbl, "Initial AC Ampl. (p-p/2)"=w611:dbl, "Final AC Ampl."=w610:dbl, "Phase (rad)"=w609:dbl, "Voltage (%)"=w608:dbl, "Gamma AC"=w607:dbl, "String"=w605:string, "Blanck"=w606:dbl)  [unwired: 1 out]
                n126 = Bundle(cluster=w603, "AC Frequency (kHz)"=w612, "Initial AC Ampl. (p-p/2)"=w611, "Final AC Ampl."=w610, "Frequency"=w598, "Phase (rad)"=w609, "Voltage (%)"=w608, "Gamma AC"=w607, "String"=w605, "Blanck"=w606) -> (w602:T18)
                n127 = Replace Array Subset(array=w601, new element=w602, index=w600) -> (w599:T15)
              }
            }
          }
          frame 1 {
            n128 = case shown="False" w614 {
              tunnel: w619 -> [w622 w626]
              tunnel: w615 -> [_ w625]
              tunnel: [w622 w624] -> w616
              tunnel: w618 -> [w621 w623]
              tunnel: [w621 w623] -> w617
              frame False {
              }
              frame True {
                n129 = Index Array(array=w626, index #1=w625, index #2=1) -> (element #1=w628:T18)  [unwired: 1 out]
                n130 = Unbundle(w628) -> ("AC Frequency (kHz)"=w637:dbl, "Initial AC Ampl. (p-p/2)"=w636:dbl, "Final AC Ampl."=w635:dbl, "Phase (rad)"=w634:dbl, "Voltage (%)"=w633:dbl, "Gamma AC"=w632:dbl, "String"=w630:string, "Blanck"=w631:dbl)  [unwired: 1 out]
                n131 = Bundle(cluster=w628, "AC Frequency (kHz)"=w637, "Initial AC Ampl. (p-p/2)"=w636, "Final AC Ampl."=w635, "Frequency"=w623, "Phase (rad)"=w634, "Voltage (%)"=w633, "Gamma AC"=w632, "String"=w630, "Blanck"=w631) -> (w627:T18)
                n132 = Replace Array Subset(array=w626, new element=w627, index=w625) -> (w624:T15)
              }
            }
          }
          frame 2 {
            n133 = Index Array(array=w643, index #1=w645, index #2=1) -> (element #1=w644:T18)  [unwired: 1 out]
            n134 = Unbundle(w644) -> ("AC Frequency (kHz)"=w654:dbl, "Initial AC Ampl. (p-p/2)"=w653:dbl, "Final AC Ampl."=w639:dbl, "Phase (rad)"=w640:dbl, "Voltage (%)"=w652:dbl, "Gamma AC"=w651:dbl, "String"=w649:string, "Blanck"=w650:dbl)  [unwired: 1 out]
            n135 = Bundle(cluster=w644, "AC Frequency (kHz)"=w654, "Initial AC Ampl. (p-p/2)"=w653, "Final AC Ampl."=w639, "Frequency"=w641, "Phase (rad)"=w640, "Voltage (%)"=w652, "Gamma AC"=w651, "String"=w649, "Blanck"=w650) -> (w642:T18)
            n136 = Replace Array Subset(array=w643, new element=w642, index=w645) -> (w638:T15)
          }
          frame 3 {
            n137 = Index Array(array=w662, index #1=w659, index #2=1) -> (element #1=w660:T18)  [unwired: 1 out]
            n138 = Unbundle(w660) -> ("AC Frequency (kHz)"=w671:dbl, "Initial AC Ampl. (p-p/2)"=w670:dbl, "Final AC Ampl."=w669:dbl, "Phase (rad)"=w668:dbl, "Voltage (%)"=w667:dbl, "Gamma AC"=w666:dbl, "String"=w665:string, "Blanck"=w656:dbl)  [unwired: 1 out]
            n139 = Bundle(cluster=w660, "AC Frequency (kHz)"=w671, "Initial AC Ampl. (p-p/2)"=w670, "Final AC Ampl."=w669, "Frequency"=w657, "Phase (rad)"=w668, "Voltage (%)"=w667, "Gamma AC"=w666, "String"=w665, "Blanck"=w656) -> (w658:T18)
            n140 = Replace Array Subset(array=w662, new element=w658, index=w659) -> (w655:T15)
          }
          frame 4 {
            n141 = Index Array(array=w679, index #1=w676, index #2=1) -> (element #1=w677:T18)  [unwired: 1 out]
            n142 = Unbundle(w677) -> ("AC Frequency (kHz)"=w678:dbl, "Initial AC Ampl. (p-p/2)"=w688:dbl, "Final AC Ampl."=w687:dbl, "Phase (rad)"=w686:dbl, "Voltage (%)"=w685:dbl, "Gamma AC"=w684:dbl, "String"=w682:string, "Blanck"=w683:dbl)  [unwired: 1 out]
            n143 = Bundle(cluster=w677, "AC Frequency (kHz)"=w678, "Initial AC Ampl. (p-p/2)"=w688, "Final AC Ampl."=w687, "Frequency"=w673, "Phase (rad)"=w686, "Voltage (%)"=w685, "Gamma AC"=w684, "String"=w682, "Blanck"=w683) -> (w674:T18)
            n144 = Replace Array Subset(array=w679, new element=w674, index=w676) -> (w672:T15)
          }
        }
        n145 = for {
          tunnel: w567 -> [w581] mode=indexing
          tunnel: w555 -> [w583] mode=indexing
          shift-right: [w580] -> w568
          shift-left: 0.0 -> [w582]
          n146 = case shown="False" w583 {
            tunnel: w582 -> [w584 w587]
            tunnel: w581 -> [_ w586]
            tunnel: [w584 w585] -> w580
            frame False {
              # "zero s"
            }
            frame True {
              n147 = Add(x=w586, y=w587) -> (x+y=w585:dbl)
            }
          }
        }
        n148 = Index Array(array=w562, index=w553) -> (element=w577:T16)
        n149 = Unbundle By Name(w577) -> ("Data Field"=w574:u32, "Output Bits"=w576:bool[], "Delay"=w565:dbl, "String"=w571:string, "OP code"=w570:u8)
        n150 = Divide(x=w568, y=1000) -> (x/y=w558:dbl)
        n151 = case shown="True" w561 {
          tunnel: w565 -> [w578 _]
          tunnel: [w578 w579] -> w564
          tunnel: w558 -> [_ w579]
          frame False {
            # "no \nchange"
          }
          frame True {
            # "match \nintevals"
          }
        }
        n152 = Bundle By Name(cluster=w577, "Data Field"=w574, "Output Bits"=w576, "Delay"=w564, "String"=w571, "OP code"=w570) -> (w575:T16)
        n153 = Replace Array Subset(array=w562, new element=w575, index=w553) -> (w572:T12)
      }
      frame 6 {
        n154 = case shown="1" w695 {
          tunnel: w697 -> [w698 w704 w710]
          tunnel: [w698 w701 w707] -> w696
          tunnel: w690 -> [_ w699 w705]
          frame 0, Default {
          }
          frame 1 {
            n155 = Unbundle By Name(w704) -> ("+6V output Voltage"=w703:dbl, "+25V output Voltage"=w702:dbl, "+25V output Current"=w700:dbl)  [unwired: 1 out]
            n156 = Bundle By Name(cluster=w704, "+6V output Voltage"=w703, "+6V output Current"=w699, "+25V output Voltage"=w702, "+25V output Current"=w700) -> (w701:T5)
          }
          frame 2 {
            n157 = Unbundle By Name(w710) -> ("+6V output Voltage"=w709:dbl, "+6V output Current"=w706:dbl, "+25V output Voltage"=w708:dbl)  [unwired: 1 out]
            n158 = Bundle By Name(cluster=w710, "+6V output Voltage"=w709, "+6V output Current"=w706, "+25V output Voltage"=w708, "+25V output Current"=w705) -> (w707:T5)
          }
        }
      }
      frame 7 {
        # "Only change frequency of SRS sine wave\n(first used for measuring trap freqs 02/2008)\nCan be modified to adjust other parameters,\nbut will need to modify SRS subVI first."
      }
    }
  }
  "PB Array of Arrays" <- w50
  "Array of 6713\nValues" <- w68
  "ArbWaveform Array\nof Channels" <- w67
  "ArbWaveform Interval Lengths" <- w66
  "changed\nquantity" <- w43
  "red mot cooling time" <- w39
  "Adiabatic Loading Waveform\nArray of Channels" <- w31
  "Power Supply Array" <- w25
  n159 = Unbundle("Waveform Change Parameters") -> ("Channel to Change"=w11:i8)  [unwired: 2 out]
  n160 = Equal?(x=0, y=w11) -> (x = y?=w15:bool)
  n161 = Equal?(x=w11, y=1) -> (x = y?=w14:bool)
  n162 = Or(x=w15, y=w14) -> (x .or. y?=w13:bool)
  n163 = And(x=w13, y=w3) -> (x .and. y?=w12:bool)
  n164 = case shown="True" w12 {
    frame False {
    }
    frame True {
      n165 = call "Display Message to User"() -> ()  [unwired: 10 in, 2 out]
    }
  }
  n166 = Bundle(cluster="SynthOutTemplate", "Table Mode On"=w3, "SynthesizerArrayofArrays"=w2) -> (→"SynthOut":T1)
  n167 = Bundle("PB parameter to change"=w54, "Column of\nData to Change\n(0, 1, 2, ....)"=w53, "Column of\nDelay to Change\n(0, 1, 2, ....)"=w52, "6713 DAC Ch\nto Change"=w51, "column for waveform\n(red mot cooling)"=w48, "column for waveform\n(dipole trap loading)"=w27) -> (→"output params to change":T9)  [unwired: 1 in]
